vi "Attocube Main.vi"() -> ()   [LabVIEW 2013]
panel:
  out "last move time":timestamp
  out "axis 1:\nCurrent position [µm/°/m°] 2":dbl(knob) scale=65.0..270.0 scale format="%#_3p"
  out "axis 1:\nCurrent position (°)":dbl format="%.4f"
  in  "set static amplitude\nwhen moving":bool
  in  "static amplitude (mV)":dbl=2.0 min=0.001 max=2.0 format="%#_13g"
  in  "both axes: Output":bool caption="both axes:\nOutput"
  in  "axis 2:\nStop moving":bool
  in  "axis 1:\nStop moving":bool
  in  "Remote mode":bool
  in  "axis 2:\nstop detection":bool
  in  "axis 1:\nstop detection":bool
  in  "axis 2:\nOutput":bool
  in  "axis 1:\ncontrol mode":enum16{"speed", "amplitude", "step size"}(ring)=enum."amplitude"
  in  "axis 2:\ncontrol mode":enum16{"speed", "amplitude", "step size"}(ring)=enum."amplitude"
  in  "axis 1:\nOutput":bool
  out "axis 2:\nStepWidth":i32=38 format="%.0fnm"
  out "axis 1:\nStepWidth":i32 format="%.0fnm"
  out "axis 2:\nspeed (°/s)":i32=31
  out "axis 1:\nspeed (°/s)":i32
  out "axis 2:\nCapacitance":i32=2486 format="%.0fnF"
  out "axis 1:\nCapacitance":i32=2534 format="%.0fnF"
  in  "axis 2:\ncap. measure":bool
  in  "axis 1:\ncap. measure":bool
  out "axis 2:\nCurrent position [µm/°/m°] 2":dbl(knob) scale=5.0..320.0
  in  "axis 2:\nFrequency [Hz]":i32=800 min=0 max=20000 format="%.0fHz"
  in  "axis 1:\nFrequency [Hz]":i32=800 min=0 max=20000 format="%.0fHz"
  in  "axis 2:\nDCLevel [V]":dbl min=0.0 max=140.0 step=0.001 format="%.3f"
  in  "axis 1:\nDCLevel [V]":dbl min=0.0 max=140.0 step=0.001 format="%.3f"
  in  "axis 2:\nAmplitude [V]":dbl=35.0 min=0.0 max=150.0 format="%.3gV"
  in  "axis 1:\nAmplitude [V]":dbl=40.0 min=0.0 max=150.0 format="%.3gV"
  in  "axis 2:\ncontinuous back":bool
  in  "axis 2:\ncontinuous fwd":bool
  in  "axis 1:\ncontinuous back":bool
  in  "axis 1:\ncontinuous fwd":bool
  in  "axis 2:\nsingle step fwd":bool
  in  "axis 2:\nsingle step back":bool
  in  "axis 1:\nsingle step back":bool
  in  "axis 1:\nsingle step fwd":bool
  in  "axis 2:\nsp position °":dbl=78.5 min=5.0 max=320.0 format="%.4g"
  in  "axis 2:\nsp rot count":i32
  in  "axis 1:\nsp rot count":i32
  in  "axis 1:\nsp position °":dbl=167.0 min=65.0 max=270.0 format="%.4g"
  in  "axis 2:\nAbsolute":bool
  in  "axis 2:\nRelative":bool
  in  "axis 1:\nRelative":bool
  in  "axis 1:\nAbsolute":bool
  in  "axis 1: \nTarget GND":bool
  in  "axis 1:\nSingle Circle Mode":bool
  in  "axis 2:\nSingle Circle Mode":bool
  in  "axis 2: \nTarget GND":bool
  out "axis 2:\npositioner status":T1
  out "axis 2:\nCurrent position (°)":dbl format="%.4f"
  out "axis 2:\nrot. count":i32
  out "axis 1:\npositioner status":T1
  out "axis 1:\nrot. count":i32
  out "handle":i32=5
  in  "OK":bool
  # "Axis 1: large axis"
  # "Axis 2: small axis"
  # "Notes: \n\n***Switch controller to ground (output=false) before connecting the rotator and while cooling down/warming up***\n\nAxis 1 (large axis): Position is limited by physical stops to angles from 65° to 270°\n\nAxis 2 (small axis): Encoded positions are limited to angles from 5° to 320°, not physically limited to one rotation.  Keep single circle mode OFF to limit the rotation count to zero and protect the wiring from over-rotating.\n\nStatic Amplitude: Sets the voltage applied to the resitive readout system.  Range: 0.001 V to 2V.  Higher voltages enhace the sensitivity but lower voltages minimize heat dissipation for low temperature applications.\n\nAbsolute: positioner travels from its current position to      the target position.\n\nTarget Ground: positioner will be grounded when the target position is reached.\n\nSingle circle mode: If OFF absolute and relative positioning are only allowed up to a full circle, keeps rot count at zero.\n\nOutput: When checked, the repective axis output is enabled.  Deactivating sets the axis to GND\n\nControl mode: \n     amplitude: individual steps of the piezo are definied by        the amplitude.  Driven in open-loop mode, travel speed and step width may vary\n     speed: feedback enables a constant travel speed by closed-loop control of the amplitude and frequency.  Speed is set by adjusting the amplitude and/or frequency values.\n     step width: Step size in controlled to a constant value.  Amplitude is closed-loop controlled.  Step width is set by adjusting the amplitude"
  # "Automatic Positioning"
  # "Automatic Positioning"
  # "Manual Positioning"
  # "Manual Positioning"
  # "Move Single Step"
  # "Move Single Step"
  # "Move Continuous"
  # "Move Continuous"
  # "Capacitance Measurement"
  # "Capacitance Measurement"
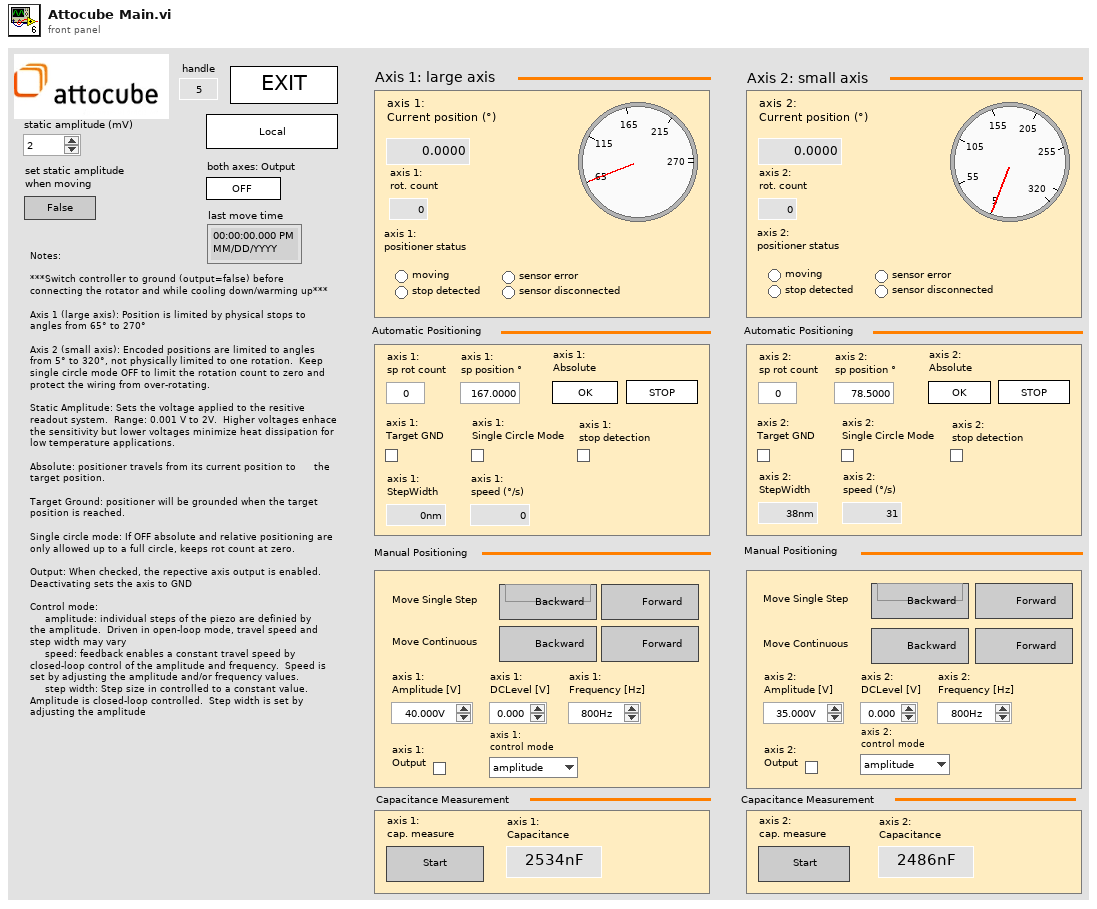
[diagram p1: front panel]
types:
  T1 = cluster{"moving":bool, "stop detected":bool, "sensor error":bool, "sensor disconnected":bool}
  T2 = enum32{"invalid app kind", "Development System", "Run Time System", "Student Edition", "Embedded LabVIEW", "Evaluation", "Custom"}
  T3 = enum32{"Invalid", "Standard", "Closed", "Hidden", "Minimized", "Maximized"}
  T4 = cluster{"axis 1: Absolute":bool, "axis 2: Absolute":bool, "axis 1: Stop moving":bool, "axis 2: Stop moving":bool, "axis 1: Output":bool, "axis 2: Output":bool, "set static amplitude\nwhen moving":bool}
  T5 = cluster{"axis 1: Amplitude [V]":dbl, "axis 2: Amplitude [V]":dbl, "axis 1: DCLevel [V]":dbl, "axis 2: DCLevel [V]":dbl, "axis 1: Frequency [Hz]":dbl, "axis 2: Frequency [Hz]":dbl, "axis 1: sp position °":dbl, "axis 2: sp position °":dbl, "axis 1: sp rot count":dbl, "axis 2: sp rot count":dbl}
  T6 = cluster{"error ":bool, "error number":i32, "error code":string}
  T7 = cluster{"Core":cluster{"Current VI Reference":refnum<vi>, "Close Panel on Exit?":bool}, "handle":i32}
  T8 = cluster{"Current VI Reference":refnum<vi>, "Close Panel on Exit?":bool}
  T9 = cluster{"axis 1: Current position (°)":dbl, "axis 2: Current position (°)":dbl, "axis 1: rot. count":dbl, "axis 2: rot. count":dbl, "axis 1: StepWidth":dbl, "axis 2: StepWidth":dbl, "axis 1: speed (°/s)":dbl, "axis 2: speed (°/s)":dbl, "axis 1: positioner status":cluster{"moving":bool, "stop detected":bool, "sensor error":bool, "sensor disconnected":bool}, "axis 2: positioner status":cluster{"moving":bool, "stop detected":bool, "sensor error":bool, "sensor disconnected":bool}}
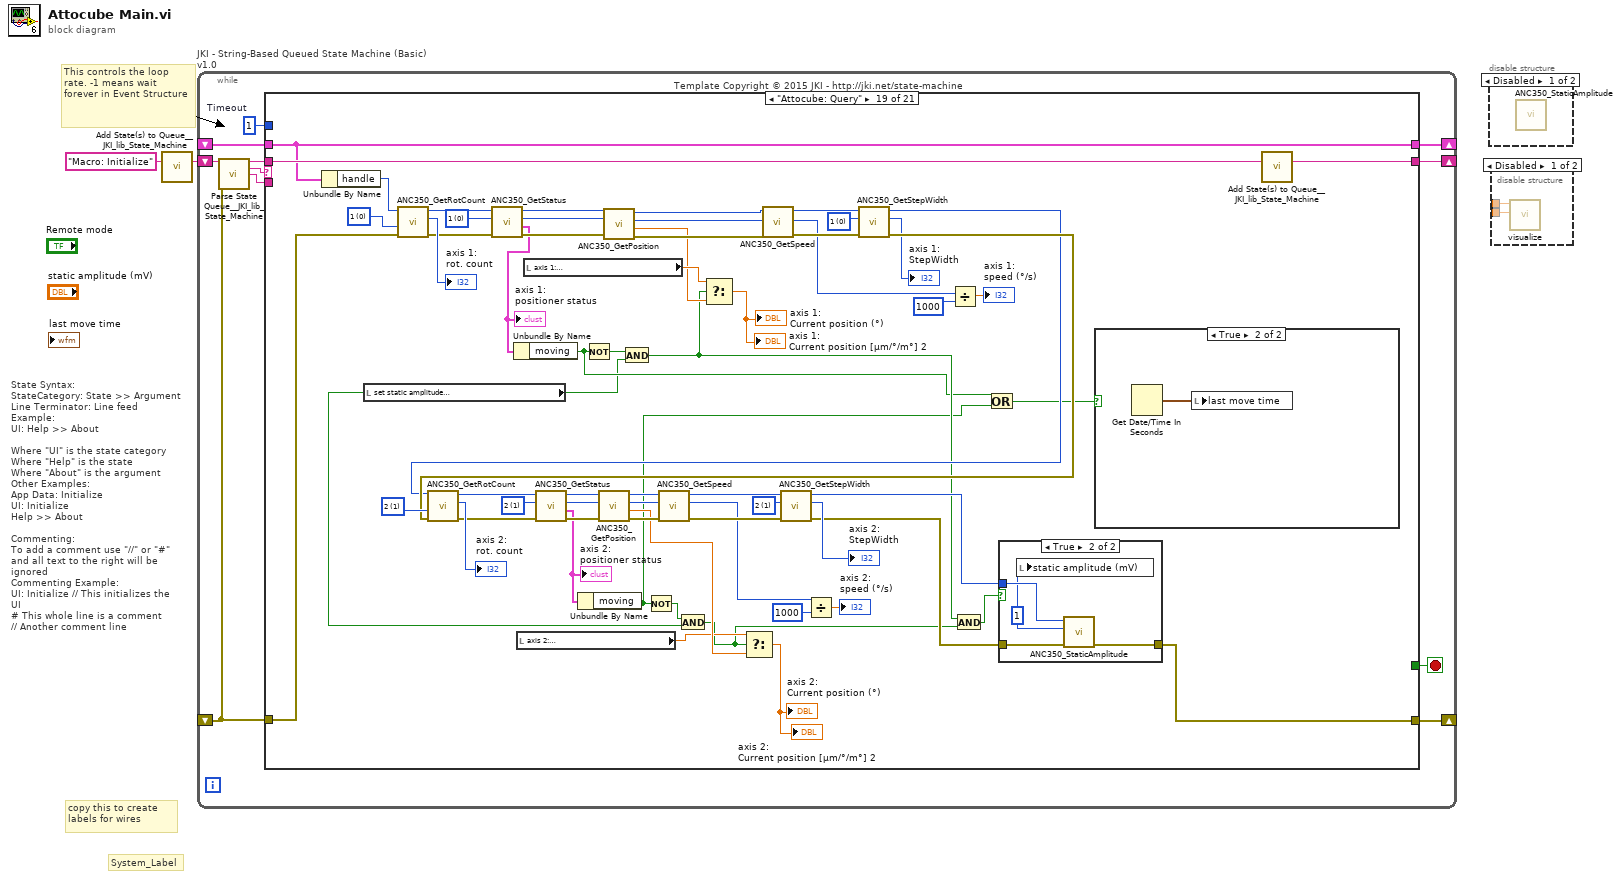
[diagram p0: block diagram]
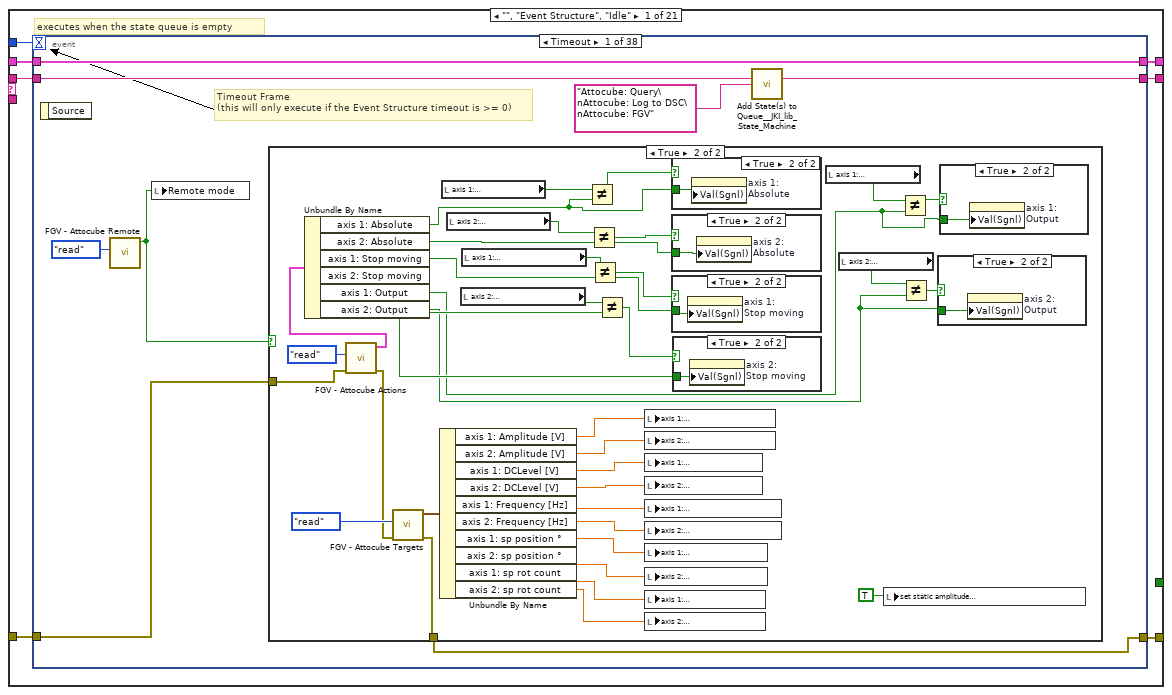
[diagram p4: hidden frame]
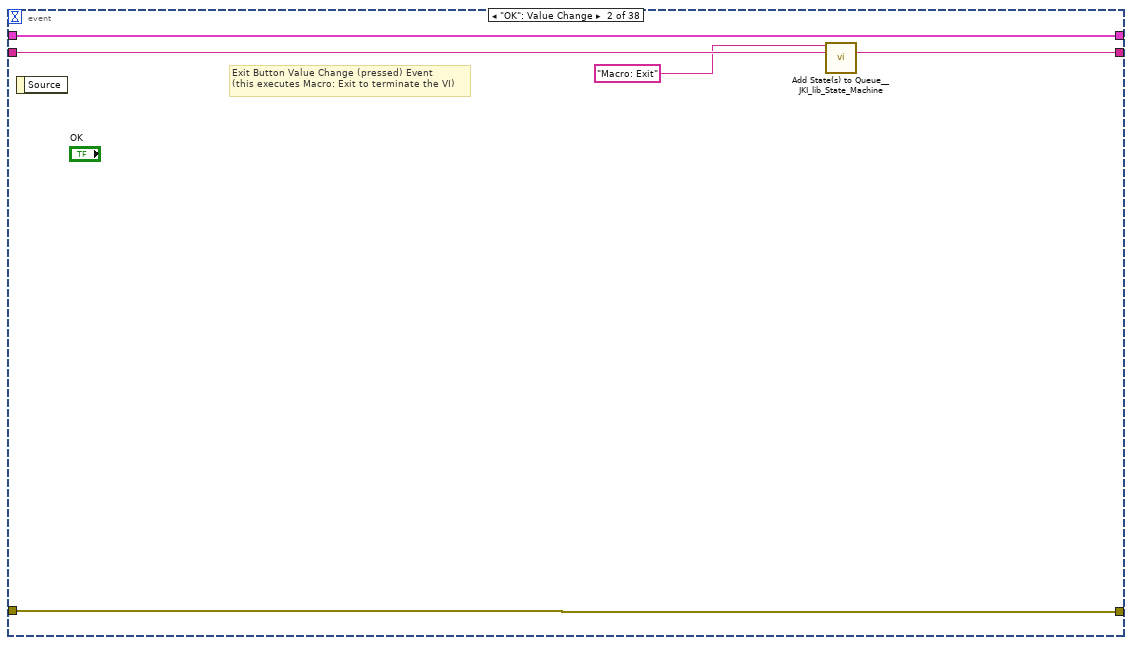
[diagram p12: hidden frame]
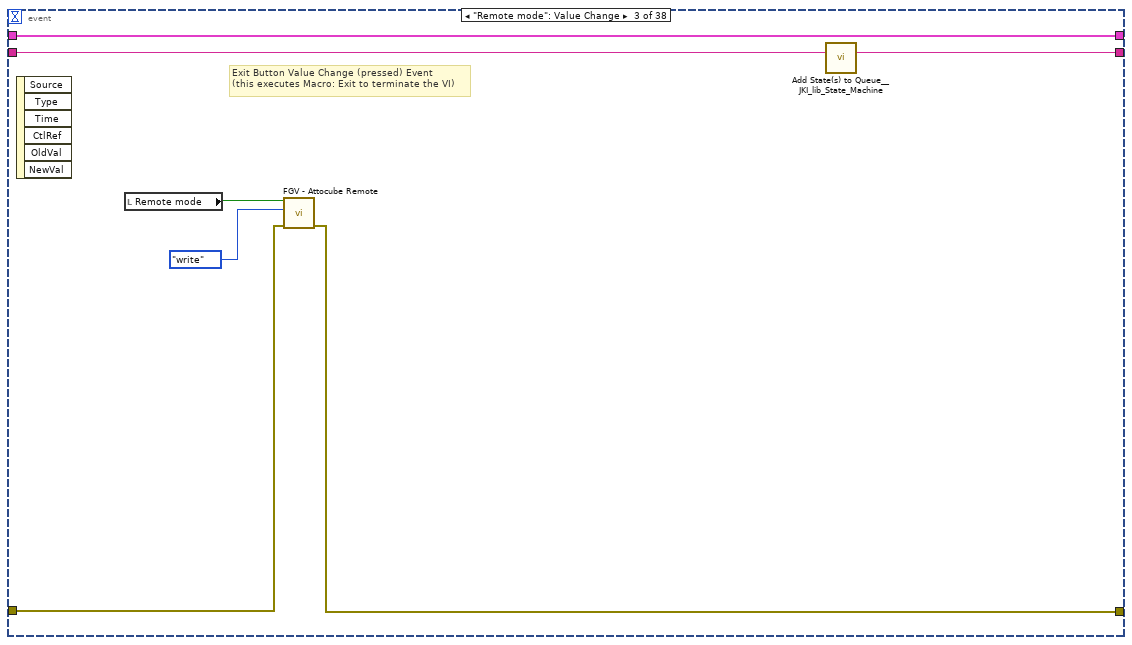
[diagram p13: hidden frame]
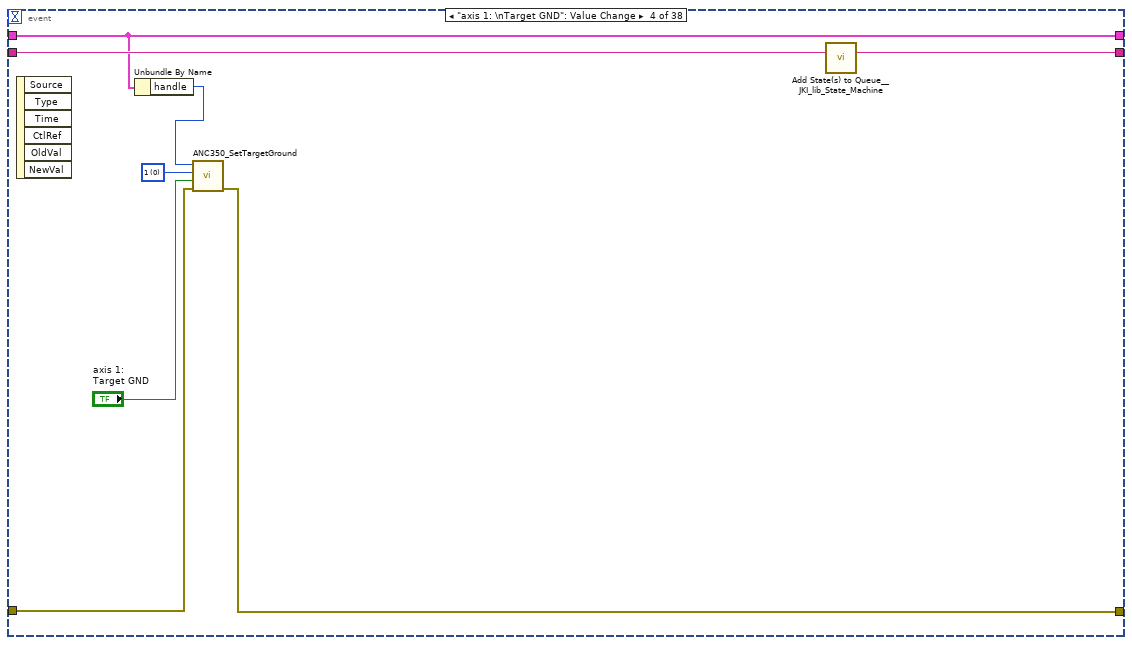
[diagram p14: hidden frame]
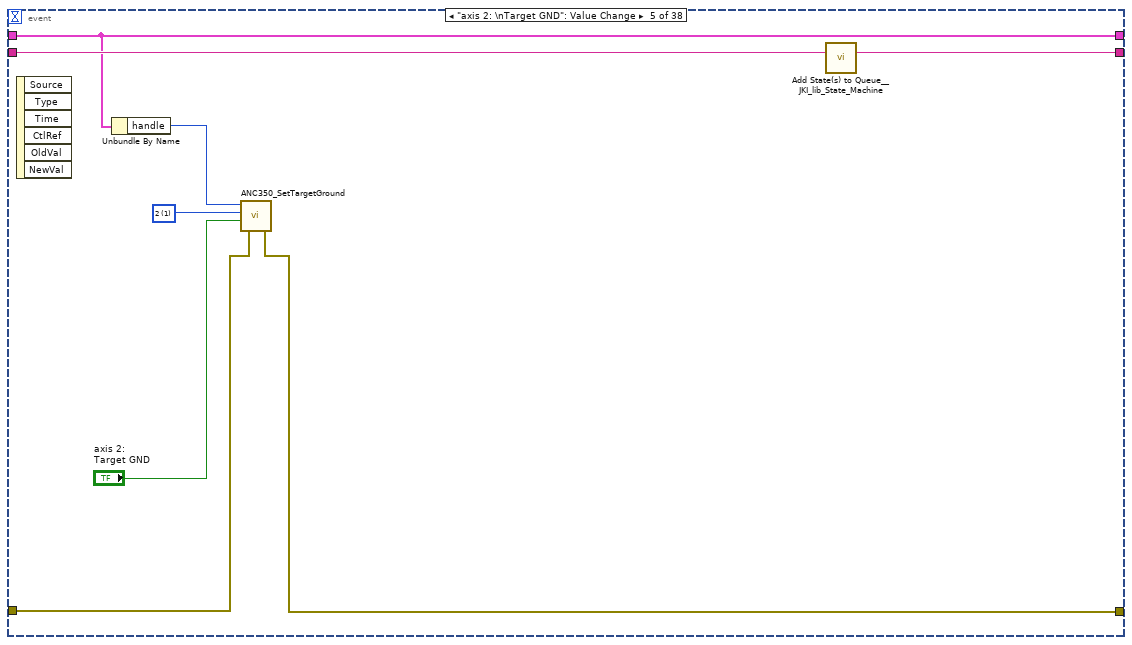
[diagram p15: hidden frame]
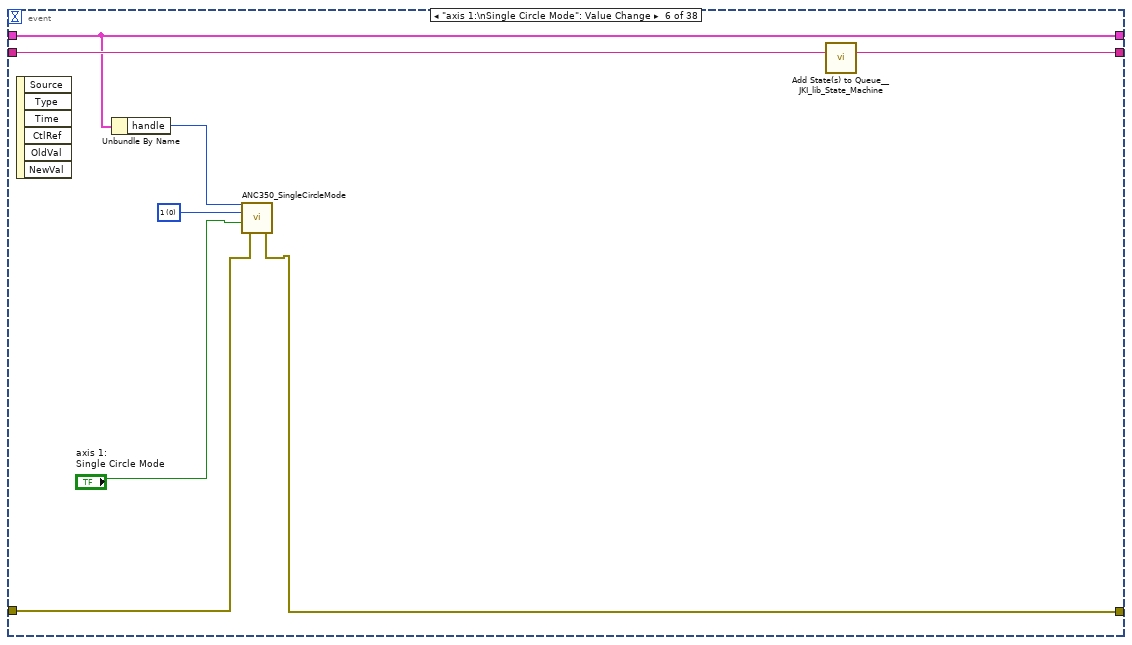
[diagram p16: hidden frame]
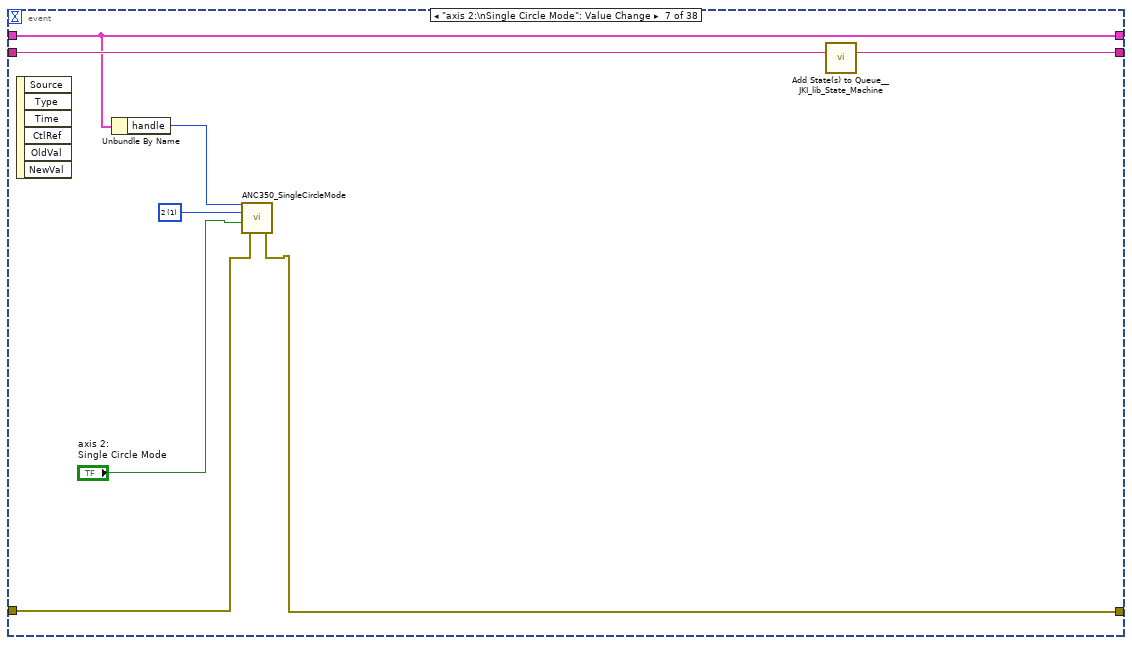
[diagram p17: hidden frame]
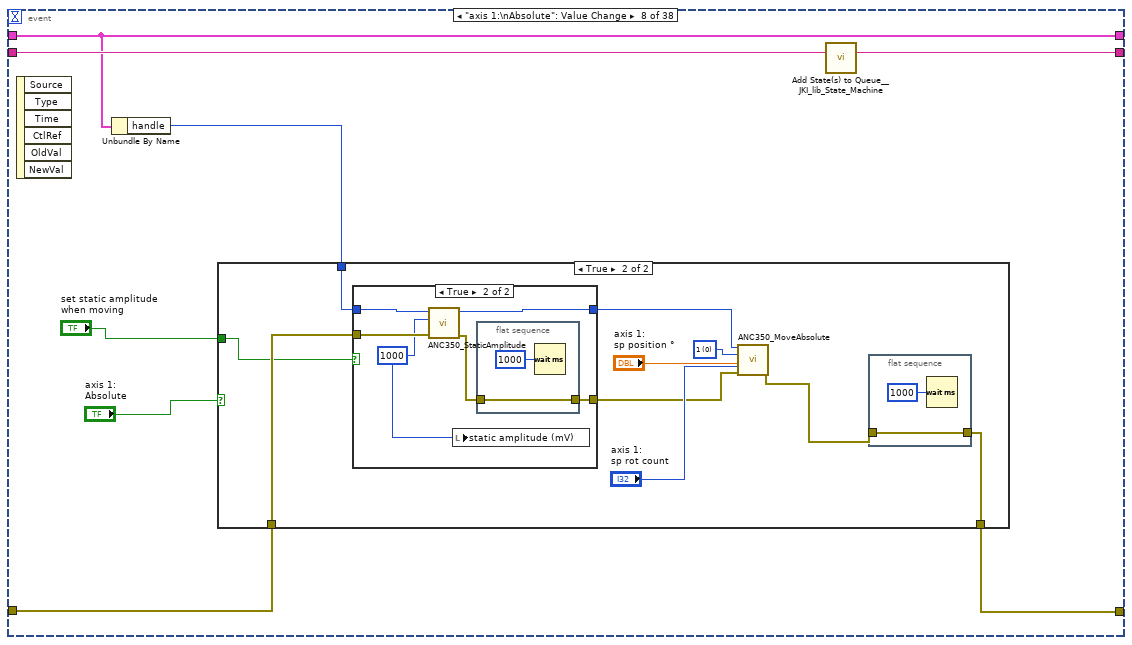
[diagram p18: hidden frame]
diagram:
  # "State Syntax:\nStateCategory: State >> Argument\nLine Terminator: Line feed\nExample:\nUI: Help >> About\n\nWhere \"UI\" is the state category\nWhere \"Help\" is the state\nWhere \"About\" is the argument\nOther Examples:\nApp Data: Initialize\nUI: Initialize\nHelp >> About\n\nCommenting:\nTo add a comment use \"//\" or \"#\" and all text to the right will be ignored\nCommenting Example:\nUI: Initialize // This initializes the UI\n# This whole line is a comment\n// Another comment line"
  # "copy this to create labels for wires"
  # "This controls the loop rate. -1 means wait forever in Event Structure"
  # "System_Label"
  n1 = call <vilib>:"Add State(s) to Queue__JKI_lib_State_Machine.vi"("State(s) in (\"\")"="Macro: Initialize") -> ("States Out"=w2:string)  [unwired: 14 in]
  n2 = while "JKI - String-Based Queued State Machine (Basic) v1.0" {
    shift-right: [w7] -> _
    shift-left: _ -> [w6]
    shift-right: [w3] -> _
    shift-left: _ -> [w4]
    shift-right: [w9] -> _
    shift-left: w2 -> [w10]
    stop <- w8 stop-if-true
    w5 = 1  # Timeout
    # "Template Copyright © 2015 JKI - http://jki.net/state-machine"
    n3 = call <vilib>:"Parse State Queue__JKI_lib_State_Machine.vi"("State Queue"=w10, "Error In (no error)"=w4) -> ("Remaining States"=w12:string, "Current State"=w13:string, "Arguments"=w11:string)  [unwired: 11 in]
    n4 = case shown="\"Attocube: Query\"" w13 {
      selector: w13 -> [_ _ w500 _ _ _ _ _ _ _ _ _ _ _ _ _ _ _ _ _ _]
      tunnel: w12 -> [w20 w499 w504 w522 w528 w533 w537 w543 w549 w553 w564 w575 w586 w612 w617 w643 w647 w655 w721 w782 w831]
      tunnel: w11 -> [_ _ _ _ _ _ _ _ _ _ _ w570 w580 _ _ _ _ _ _ _ _]
      tunnel: w6 -> [w18 w496 w502 w513 w525 w531 w534 _ w544 w550 w562 w573 w582 w609 w614 w641 w644 w653 w719 w780 w829]
      tunnel: w4 -> [w16 w497 w505 w519 w524 w530 w535 w540 w546 w551 w561 w572 w584 w610 w615 w631 w645 _ w718 w735 w824]
      tunnel: [w19 w498 w503 w521 w527 w532 w536 w542 w548 w552 w563 w574 w585 w611 w616 w642 w646 w654 w720 w781 w830] -> w9
      tunnel: [_ _ _ _ _ TRUE _ _ _ _ _ _ _ _ _ _ _ _ _ _ _] -> w8
      tunnel: [w15 w496 w502 w520 w525 w531 w534 w541 w544 w550 w562 w573 w582 w609 w614 w641 w644 w652 w719 w780 w829] -> w7
      tunnel: w5 -> [w14 _ _ _ _ _ _ _ _ _ _ _ _ _ _ _ _ _ _ _ _]
      tunnel: [w17 w497 w506 w519 errorcluster {"status"=FALSE, "code"=0, "source"=""} ("error out") w530 w535 w540 w545 w551 w561 w571 w583 w610 w615 w634 w645 w649 w668 w735 w787] -> w3
      frame "", "Event Structure", "Idle" {
        # "executes when the state queue is empty"
        n5 = event shown="[0] Timeout" {
          selector: _ -> [_ _ _ _ _ _ _ _ _ _ _ _ _ _ _ _ _ _ _ _ _ _ _ _ _ _ _ _ _ _ _ _ _ _ _ _ _ _]
          dyn-events: _ -> [_ _ _ _ _ _ _ _ _ _ _ _ _ _ _ _ _ _ _ _ _ _ _ _ _ _ _ _ _ _ _ _ _ _ _ _ _ _]
          timeout: w14 -> [_ _ _ _ _ _ _ _ _ _ _ _ _ _ _ _ _ _ _ _ _ _ _ _ _ _ _ _ _ _ _ _ _ _ _ _ _ _]
          tunnel: w20 -> [w28 w76 w83 w91 w99 w107 w115 w123 w154 w184 w198 w212 w225 w238 w251 w264 w280 w296 w312 w329 w337 w345 w353 w361 w369 w377 w391 w405 w413 w421 w429 w437 w445 w453 w466 w476 w484 w495]
          tunnel: [w27 w75 w82 w90 w98 w106 w114 w122 w153 w183 w197 w211 w224 w237 w250 w263 w279 w295 w311 w328 w336 w344 w352 w360 w368 w376 w390 w404 w412 w420 w428 w436 w444 w452 w465 w475 w483 w494] -> w19
          tunnel: w18 -> [w26 w73 w81 w89 w97 w105 w113 w121 w152 w182 w196 w210 w223 w236 w249 w262 w278 w294 w310 w327 w335 w343 w351 w359 w367 w375 w389 w403 w411 w419 w427 w435 w443 w451 w464 w474 w482 w492]
          tunnel: [w21 w74 w77 w84 w94 w100 w110 w116 w149 w179 w193 w207 w220 w233 w246 w259 w275 w291 w307 w322 w331 w338 w347 w354 w363 w371 w385 w399 w407 w416 w424 w431 w439 w447 w460 w473 w479 w493] -> w17
          tunnel: w16 -> [w22 w74 w78 w85 w95 w101 w111 w119 w150 w180 w194 w208 w221 w234 w247 w260 w276 w292 w308 w323 w332 w339 w348 w355 w364 w372 w386 w400 w408 w417 w425 w432 w440 w448 w461 w473 w480 w493]
          tunnel: [w26 w73 w81 w89 w97 w105 w113 w121 w152 w182 w196 w210 w223 w236 w249 w262 w278 w294 w310 w327 w335 w343 w351 w359 w367 w375 w389 w403 w411 w419 w427 w435 w443 w451 w464 w474 w482 w492] -> w15
          event Timeout {
            # "Timeout Frame\n(this will only execute if the Event Structure timeout is >= 0)"
            n6 = event-data() -> ()  [unwired: 1 in, 1 out]
            n7 = call "FGV - Attocube Remote.vi"("Function"=enum16{"write", "read"}."read") -> ("Attocube Remote"=w23:bool)  [unwired: 5 in, 1 out]
            n8 = local write "Remote mode"(w23) -> ()
            n9 = case shown="True" w23 {
              tunnel: w22 -> [w29 w39]
              tunnel: [w29 w37] -> w21
              frame False {
              }
              frame True {
                n10 = call "FGV - Attocube Actions.vi"("error in"=w39, "Function"=enum16{"write", "read"}."read") -> ("error out"=w38:errorcluster, "Actions OUT"=w64:T4)  [unwired: 4 in]
                n11 = Unbundle By Name(w64) -> ("axis 1: Absolute"=w58:bool, "axis 2: Absolute"=w57:bool, "axis 1: Stop moving"=w53:bool, "axis 2: Stop moving"=w52:bool, "axis 1: Output"=w33:bool, "axis 2: Output"=w30:bool)
                n12 = call "FGV - Attocube Targets.vi"("error in"=w38, "Function"=enum16{"write", "read"}."read") -> ("error out"=w37:errorcluster, "Targets Out"=w50:T5)  [unwired: 4 in]
                n13 = Unbundle By Name(w50) -> ("axis 1: Amplitude [V]"=w49:dbl, "axis 2: Amplitude [V]"=w48:dbl, "axis 1: DCLevel [V]"=w47:dbl, "axis 2: DCLevel [V]"=w46:dbl, "axis 1: Frequency [Hz]"=w45:dbl, "axis 2: Frequency [Hz]"=w44:dbl, "axis 1: sp position °"=w43:dbl, "axis 2: sp position °"=w42:dbl, "axis 1: sp rot count"=w41:dbl, "axis 2: sp rot count"=w40:dbl)
                n14 = local read "axis 1:\nAbsolute"() -> (w63:bool)
                n15 = local read "axis 2:\nAbsolute"() -> (w62:bool)
                n16 = local read "axis 2:\nStop moving"() -> (w60:bool)
                n17 = local read "axis 1:\nStop moving"() -> (w61:bool)
                n18 = Not Equal?(x=w63, y=w58) -> (x != y?=w59:bool)
                n19 = Not Equal?(x=w62, y=w57) -> (x != y?=w56:bool)
                n20 = Not Equal?(x=w61, y=w53) -> (x != y?=w55:bool)
                n21 = Not Equal?(x=w60, y=w52) -> (x != y?=w54:bool)
                n22 = local write "axis 1:\nAmplitude [V]"(w49) -> ()
                n23 = local write "axis 2:\nAmplitude [V]"(w48) -> ()
                n24 = local write "axis 1:\nDCLevel [V]"(w47) -> ()
                n25 = local write "axis 2:\nDCLevel [V]"(w46) -> ()
                n26 = local write "axis 1:\nFrequency [Hz]"(w45) -> ()
                n27 = local write "axis 2:\nFrequency [Hz]"(w44) -> ()
                n28 = local write "axis 1:\nsp position °"(w43) -> ()
                n29 = local write "axis 2:\nsp position °"(w42) -> ()
                n30 = local write "axis 1:\nsp rot count"(w41) -> ()
                n31 = local write "axis 2:\nsp rot count"(w40) -> ()
                n32 = case shown="True" w59 {
                  tunnel: w58 -> [_ w71]
                  frame False {
                  }
                  frame True {
                    n33 = property on="axis 1:\nAbsolute" class="Bool (strict)"("Val(Sgnl)"=w71) -> ()  [unwired: 2 in, 2 out]
                  }
                }
                n34 = case shown="True" w56 {
                  tunnel: w57 -> [_ w70]
                  frame False {
                  }
                  frame True {
                    n35 = property on="axis 2:\nAbsolute" class="Bool (strict)"("Val(Sgnl)"=w70) -> ()  [unwired: 2 in, 2 out]
                  }
                }
                n36 = case shown="True" w55 {
                  tunnel: w53 -> [_ w69]
                  frame False {
                  }
                  frame True {
                    n37 = property on="axis 1:\nStop moving" class="Bool (strict)"("Val(Sgnl)"=w69) -> ()  [unwired: 2 in, 2 out]
                  }
                }
                n38 = case shown="True" w54 {
                  tunnel: w52 -> [_ w68]
                  frame False {
                  }
                  frame True {
                    n39 = property on="axis 2:\nStop moving" class="Bool (strict)"("Val(Sgnl)"=w68) -> ()  [unwired: 2 in, 2 out]
                  }
                }
                n40 = local read "axis 1:\nOutput"() -> (w34:bool)
                n41 = local read "axis 2:\nOutput"() -> (w31:bool)
                n42 = local write "set static amplitude\nwhen moving"(TRUE) -> ()
                n43 = Not Equal?(x=w34, y=w33) -> (x != y?=w35:bool)
                n44 = Not Equal?(x=w31, y=w30) -> (x != y?=w32:bool)
                n45 = case shown="True" w32 {
                  tunnel: w30 -> [_ w66]
                  frame False {
                  }
                  frame True {
                    n46 = property on="axis 2:\nOutput" class="Bool (strict)"("Val(Sgnl)"=w66) -> ()  [unwired: 2 in, 2 out]
                  }
                }
                n47 = case shown="True" w35 {
                  tunnel: w33 -> [_ w67]
                  frame False {
                  }
                  frame True {
                    n48 = property on="axis 1:\nOutput" class="Bool (strict)"("Val(Sgnl)"=w67) -> ()  [unwired: 2 in, 2 out]
                  }
                }
              }
            }
            n49 = call <vilib>:"Add State(s) to Queue__JKI_lib_State_Machine.vi"("State(s) in (\"\")"=w28, "State(s) at Back (\"\")"="Attocube: Query\nAttocube: Log to DSC\nAttocube: FGV" ("State(s) at Back (\"\")")) -> ("States Out"=w27:string)  [unwired: 13 in]
          }
          event "OK": Value Change {
            # "Exit Button Value Change (pressed) Event\n(this executes Macro: Exit to terminate the VI)"
            n50 = event-data() -> ()  [unwired: 1 in, 1 out]
            n51 = call <vilib>:"Add State(s) to Queue__JKI_lib_State_Machine.vi"("State(s) in Front (\"\")"="Macro: Exit", "State(s) in (\"\")"=w76) -> ("States Out"=w75:string)  [unwired: 13 in]
          }
          event "Remote mode": Value Change {
            # "Exit Button Value Change (pressed) Event\n(this executes Macro: Exit to terminate the VI)"
            n52 = event-data() -> ()  [unwired: 1 in, 6 out]
            n53 = local read "Remote mode"() -> (w80:bool)
            n54 = call "FGV - Attocube Remote.vi"("error in"=w78, "Function"=enum16{"write", "read"}."write", "Attocube Remote"=w80) -> ("error out"=w77:errorcluster)  [unwired: 3 in, 1 out]
            n55 = call <vilib>:"Add State(s) to Queue__JKI_lib_State_Machine.vi"("State(s) in (\"\")"=w83) -> ("States Out"=w82:string)  [unwired: 14 in]
          }
          event "axis 1: \nTarget GND": Value Change {
            w87 = u8 0 items=["1", "2", "3", "4", "5", "6", "7", "8", "9"] ("axis no")
            n56 = event-data() -> ()  [unwired: 1 in, 6 out]
            n57 = Unbundle By Name(w89) -> ("handle"=w88:i32)
            n58 = call "ANC350_SetTargetGround.vi"("error in"=w85, "PositionerAcIn"="axis 1: \nTarget GND", "axis no"=w87, "device handle"=w88) -> ("error out"=w84:T6)  [unwired: 2 in, 1 out]
            n59 = call <vilib>:"Add State(s) to Queue__JKI_lib_State_Machine.vi"("State(s) in (\"\")"=w91) -> ("States Out"=w90:string)  [unwired: 14 in]
          }
          event "axis 2: \nTarget GND": Value Change {
            w93 = u8 1 items=["1", "2", "3", "4", "5", "6", "7", "8", "9"] ("axis no")
            n60 = event-data() -> ()  [unwired: 1 in, 6 out]
            n61 = Unbundle By Name(w97) -> ("handle"=w96:i32)
            n62 = call "ANC350_SetTargetGround.vi"("error in"=w95, "PositionerAcIn"="axis 2: \nTarget GND", "axis no"=w93, "device handle"=w96) -> ("error out"=w94:T6)  [unwired: 2 in, 1 out]
            n63 = call <vilib>:"Add State(s) to Queue__JKI_lib_State_Machine.vi"("State(s) in (\"\")"=w99) -> ("States Out"=w98:string)  [unwired: 14 in]
          }
          event "axis 1:\nSingle Circle Mode": Value Change {
            w103 = u8 0 items=["1", "2", "3", "4", "5", "6", "7", "8", "9"] ("axis no")
            n64 = event-data() -> ()  [unwired: 1 in, 6 out]
            n65 = Unbundle By Name(w105) -> ("handle"=w104:i32)
            n66 = call "ANC350_SingleCircleMode.vi"("error in"=w101, "enable"="axis 1:\nSingle Circle Mode", "axis no"=w103, "device handle"=w104) -> ("error out"=w100:T6)  [unwired: 2 in, 1 out]
            n67 = call <vilib>:"Add State(s) to Queue__JKI_lib_State_Machine.vi"("State(s) in (\"\")"=w107) -> ("States Out"=w106:string)  [unwired: 14 in]
          }
          event "axis 2:\nSingle Circle Mode": Value Change {
            w108 = u8 1 items=["1", "2", "3", "4", "5", "6", "7", "8", "9"] ("axis no")
            n68 = event-data() -> ()  [unwired: 1 in, 6 out]
            n69 = Unbundle By Name(w113) -> ("handle"=w112:i32)
            n70 = call "ANC350_SingleCircleMode.vi"("error in"=w111, "enable"="axis 2:\nSingle Circle Mode", "axis no"=w108, "device handle"=w112) -> ("error out"=w110:T6)  [unwired: 2 in, 1 out]
            n71 = call <vilib>:"Add State(s) to Queue__JKI_lib_State_Machine.vi"("State(s) in (\"\")"=w115) -> ("States Out"=w114:string)  [unwired: 14 in]
          }
          event "axis 1:\nAbsolute": Value Change {
            n72 = event-data() -> ()  [unwired: 1 in, 6 out]
            n73 = Unbundle By Name(w121) -> ("handle"=w120:i32)
            n74 = case shown="True" "axis 1:\nAbsolute" {
              tunnel: w120 -> [_ w131]
              tunnel: w119 -> [w124 w129]
              tunnel: "set static amplitude\nwhen moving" -> [_ w127]
              tunnel: [w124 w125] -> w116
              frame False {
              }
              frame True {
                w134 = u8 0 items=["1", "2", "3", "4", "5", "6", "7", "8", "9"] ("axis no")
                n75 = case shown="True" w127 {
                  tunnel: w131 -> [w138 w144]
                  tunnel: [w138 w143] -> w130
                  tunnel: w129 -> [w137 w142]
                  tunnel: [w137 w140] -> w128
                  frame False {
                  }
                  frame True {
                    w139 = 1000 ("static amplitude")
                    n76 = call "ANC350_StaticAmplitude.vi"("error in"=w142, "static amplitude"=w139, "device handle"=w144) -> ("error out"=w141:T6, "device handle Out"=w143:i32)  [unwired: 3 in]
                    n77 = local write "static amplitude (mV)"(w139) -> ()
                    n78 = flat-sequence {
                      tunnel: [w146] -> w140
                      tunnel: w141 -> [w146]
                      frame #0 {
                        n79 = Wait (ms)(milliseconds to wait=u32 1000) -> ()  [unwired: 1 out]
                      }
                    }
                  }
                }
                n80 = call "ANC350_MoveAbsolute.vi"("device handle"=w130, "axis no"=w134, "absoluteposition [µm/°/m°]"="axis 1:\nsp position °", "rot count"="axis 1:\nsp rot count", "error in"=w128) -> ("error out"=w126:T6)  [unwired: 9 in, 1 out]
                n81 = flat-sequence {
                  tunnel: [w136] -> w125
                  tunnel: w126 -> [w136]
                  frame #0 {
                    n82 = Wait (ms)(milliseconds to wait=u32 1000) -> ()  [unwired: 1 out]
                  }
                }
              }
            }
            n83 = call <vilib>:"Add State(s) to Queue__JKI_lib_State_Machine.vi"("State(s) in (\"\")"=w123) -> ("States Out"=w122:string)  [unwired: 14 in]
          }
          event "axis 2:\nAbsolute": Value Change {
            n84 = event-data() -> ()  [unwired: 1 in, 6 out]
            n85 = local read "set static amplitude\nwhen moving"() -> (w147:bool)
            n86 = Unbundle By Name(w152) -> ("handle"=w151:i32)
            n87 = case shown="True" "axis 2:\nAbsolute" {
              tunnel: w151 -> [_ w162]
              tunnel: w150 -> [w155 w160]
              tunnel: [w155 w156] -> w149
              tunnel: w147 -> [_ w158]
              frame False {
              }
              frame True {
                w165 = u8 1 items=["1", "2", "3", "4", "5", "6", "7", "8", "9"] ("axis no")
                n88 = case shown="True" w158 {
                  tunnel: w162 -> [w169 w175]
                  tunnel: [w169 w174] -> w161
                  tunnel: w160 -> [w168 w173]
                  tunnel: [w168 w171] -> w159
                  frame False {
                  }
                  frame True {
                    w170 = 1000 ("static amplitude")
                    n89 = local write "static amplitude (mV)"(w170) -> ()
                    n90 = call "ANC350_StaticAmplitude.vi"("error in"=w173, "static amplitude"=w170, "device handle"=w175) -> ("error out"=w172:T6, "device handle Out"=w174:i32)  [unwired: 3 in]
                    n91 = flat-sequence {
                      tunnel: [w177] -> w171
                      tunnel: w172 -> [w177]
                      frame #0 {
                        n92 = Wait (ms)(milliseconds to wait=u32 1000) -> ()  [unwired: 1 out]
                      }
                    }
                  }
                }
                n93 = call "ANC350_MoveAbsolute.vi"("device handle"=w161, "axis no"=w165, "absoluteposition [µm/°/m°]"="axis 2:\nsp position °", "rot count"="axis 2:\nsp rot count", "error in"=w159) -> ("error out"=w157:T6)  [unwired: 9 in, 1 out]
                n94 = flat-sequence {
                  tunnel: [w167] -> w156
                  tunnel: w157 -> [w167]
                  frame #0 {
                    n95 = Wait (ms)(milliseconds to wait=u32 1000) -> ()  [unwired: 1 out]
                  }
                }
              }
            }
            n96 = call <vilib>:"Add State(s) to Queue__JKI_lib_State_Machine.vi"("State(s) in (\"\")"=w154) -> ("States Out"=w153:string)  [unwired: 14 in]
          }
          event "axis 1:\nRelative": Value Change {
            n97 = event-data() -> ()  [unwired: 1 in, 6 out]
            n98 = disable-structure shown="Disabled" {
              frame Disabled {
              }
              frame Enabled {
              }
            }
            n99 = Unbundle By Name(w182) -> ("handle"=w181:i32)
            n100 = case shown="True" FALSE {
              tunnel: w181 -> [_ w191]
              tunnel: w180 -> [w185 w189]
              tunnel: [w185 w186] -> w179
              frame False {
              }
              frame True {
                w190 = u8 0 items=["1", "2", "3", "4", "5", "6", "7", "8", "9"] ("axis no")
                n101 = local read "axis 1:\nsp position °"() -> (w188:dbl)
                n102 = local read "axis 1:\nsp rot count"() -> (w187:i32)
                n103 = call "ANC350_MoveRelative.vi"("device handle"=w191, "axis no"=w190, "distance [µm/°/m°]"=w188, "rot count"=w187, "error in"=w189) -> ("error out"=w186:T6)  [unwired: 9 in, 1 out]
              }
            }
            n104 = call <vilib>:"Add State(s) to Queue__JKI_lib_State_Machine.vi"("State(s) in (\"\")"=w184) -> ("States Out"=w183:string)  [unwired: 14 in]
          }
          event "axis 2:\nRelative": Value Change {
            n105 = event-data() -> ()  [unwired: 1 in, 6 out]
            n106 = disable-structure shown="Disabled" {
              frame Disabled {
              }
              frame Enabled {
              }
            }
            n107 = Unbundle By Name(w196) -> ("handle"=w195:i32)
            n108 = case shown="True" FALSE {
              tunnel: w195 -> [_ w205]
              tunnel: w194 -> [w199 w203]
              tunnel: [w199 w202] -> w193
              frame False {
              }
              frame True {
                w204 = u8 1 items=["1", "2", "3", "4", "5", "6", "7", "8", "9"] ("axis no")
                n109 = local read "axis 2:\nsp position °"() -> (w201:dbl)
                n110 = local read "axis 2:\nsp rot count"() -> (w200:i32)
                n111 = call "ANC350_MoveRelative.vi"("device handle"=w205, "axis no"=w204, "distance [µm/°/m°]"=w201, "rot count"=w200, "error in"=w203) -> ("error out"=w202:T6)  [unwired: 9 in, 1 out]
              }
            }
            n112 = call <vilib>:"Add State(s) to Queue__JKI_lib_State_Machine.vi"("State(s) in (\"\")"=w198) -> ("States Out"=w197:string)  [unwired: 14 in]
          }
          event "axis 1:\nsingle step fwd": Value Change {
            n113 = event-data() -> ()  [unwired: 1 in, 6 out]
            n114 = Unbundle By Name(w210) -> ("handle"=w209:i32)
            n115 = case shown="True" "axis 1:\nsingle step fwd" {
              tunnel: w209 -> [_ w218]
              tunnel: w208 -> [w213 w215]
              tunnel: [w213 w214] -> w207
              frame False {
              }
              frame True {
                w217 = u8 0 items=["1", "2", "3", "4", "5", "6", "7", "8", "9"] ("axis no")
                n116 = call "ANC350_MoveSingleStep.vi"("error in"=w215, "single step direction"=FALSE, "axis no"=w217, "device handle"=w218) -> ("error out"=w214:T6)  [unwired: 2 in, 1 out]
              }
            }
            n117 = call <vilib>:"Add State(s) to Queue__JKI_lib_State_Machine.vi"("State(s) in (\"\")"=w212) -> ("States Out"=w211:string)  [unwired: 14 in]
          }
          event "axis 1:\nsingle step back": Value Change {
            n118 = event-data() -> ()  [unwired: 1 in, 6 out]
            n119 = Unbundle By Name(w223) -> ("handle"=w222:i32)
            n120 = case shown="True" "axis 1:\nsingle step back" {
              tunnel: w222 -> [_ w231]
              tunnel: w221 -> [w226 w228]
              tunnel: [w226 w227] -> w220
              frame False {
              }
              frame True {
                w230 = u8 0 items=["1", "2", "3", "4", "5", "6", "7", "8", "9"] ("axis no")
                n121 = call "ANC350_MoveSingleStep.vi"("error in"=w228, "single step direction"=TRUE, "axis no"=w230, "device handle"=w231) -> ("error out"=w227:T6)  [unwired: 2 in, 1 out]
              }
            }
            n122 = call <vilib>:"Add State(s) to Queue__JKI_lib_State_Machine.vi"("State(s) in (\"\")"=w225) -> ("States Out"=w224:string)  [unwired: 14 in]
          }
          event "axis 2:\nsingle step fwd": Value Change {
            n123 = event-data() -> ()  [unwired: 1 in, 6 out]
            n124 = Unbundle By Name(w236) -> ("handle"=w235:i32)
            n125 = case shown="True" "axis 2:\nsingle step fwd" {
              tunnel: w235 -> [_ w244]
              tunnel: w234 -> [w239 w241]
              tunnel: [w239 w240] -> w233
              frame False {
              }
              frame True {
                w243 = u8 1 items=["1", "2", "3", "4", "5", "6", "7", "8", "9"] ("axis no")
                n126 = call "ANC350_MoveSingleStep.vi"("error in"=w241, "single step direction"=FALSE, "axis no"=w243, "device handle"=w244) -> ("error out"=w240:T6)  [unwired: 2 in, 1 out]
              }
            }
            n127 = call <vilib>:"Add State(s) to Queue__JKI_lib_State_Machine.vi"("State(s) in (\"\")"=w238) -> ("States Out"=w237:string)  [unwired: 14 in]
          }
          event "axis 2:\nsingle step back": Value Change {
            n128 = event-data() -> ()  [unwired: 1 in, 6 out]
            n129 = Unbundle By Name(w249) -> ("handle"=w248:i32)
            n130 = case shown="False" "axis 2:\nsingle step back" {
              tunnel: w248 -> [_ w257]
              tunnel: w247 -> [w252 w254]
              tunnel: [w252 w253] -> w246
              frame False {
              }
              frame True {
                w256 = u8 1 items=["1", "2", "3", "4", "5", "6", "7", "8", "9"] ("axis no")
                n131 = call "ANC350_MoveSingleStep.vi"("error in"=w254, "single step direction"=TRUE, "axis no"=w256, "device handle"=w257) -> ("error out"=w253:T6)  [unwired: 2 in, 1 out]
              }
            }
            n132 = call <vilib>:"Add State(s) to Queue__JKI_lib_State_Machine.vi"("State(s) in (\"\")"=w251) -> ("States Out"=w250:string)  [unwired: 14 in]
          }
          event "axis 1:\ncontinuous fwd": Value Change {
            n133 = event-data() -> ()  [unwired: 1 in, 6 out]
            n134 = Unbundle By Name(w262) -> ("handle"=w261:i32)
            n135 = case shown="False" "axis 1:\ncontinuous fwd" {
              tunnel: w261 -> [w268 w273]
              tunnel: w260 -> [w267 w271]
              tunnel: [w266 w270] -> w259
              frame False {
                w265 = u8 0 items=["1", "2", "3", "4", "5", "6", "7", "8", "9"] ("axis no")
                n136 = call "ANC350_StopMoving.vi"("error in"=w267, "axis no"=w265, "device handle"=w268) -> ("error out"=w266:T6)  [unwired: 3 in, 1 out]
              }
              frame True {
                w272 = u8 0 items=["1", "2", "3", "4", "5", "6", "7", "8", "9"] ("axis no")
                n137 = call "ANC350_MoveContinuous.vi"("error in"=w271, "step direction"=FALSE ("single step direction"), "axis no"=w272, "device handle"=w273) -> ("error out"=w270:T6)  [unwired: 2 in, 1 out]
              }
            }
            n138 = call <vilib>:"Add State(s) to Queue__JKI_lib_State_Machine.vi"("State(s) in (\"\")"=w264) -> ("States Out"=w263:string)  [unwired: 14 in]
          }
          event "axis 1:\ncontinuous back": Value Change {
            n139 = event-data() -> ()  [unwired: 1 in, 6 out]
            n140 = Unbundle By Name(w278) -> ("handle"=w277:i32)
            n141 = case shown="True" "axis 1:\ncontinuous back" {
              tunnel: w277 -> [w284 w289]
              tunnel: w276 -> [w283 w287]
              tunnel: [w282 w286] -> w275
              frame False {
                w281 = u8 0 items=["1", "2", "3", "4", "5", "6", "7", "8", "9"] ("axis no")
                n142 = call "ANC350_StopMoving.vi"("error in"=w283, "axis no"=w281, "device handle"=w284) -> ("error out"=w282:T6)  [unwired: 3 in, 1 out]
              }
              frame True {
                w288 = u8 0 items=["1", "2", "3", "4", "5", "6", "7", "8", "9"] ("axis no")
                n143 = call "ANC350_MoveContinuous.vi"("error in"=w287, "step direction"=TRUE ("single step direction"), "axis no"=w288, "device handle"=w289) -> ("error out"=w286:T6)  [unwired: 2 in, 1 out]
              }
            }
            n144 = call <vilib>:"Add State(s) to Queue__JKI_lib_State_Machine.vi"("State(s) in (\"\")"=w280) -> ("States Out"=w279:string)  [unwired: 14 in]
          }
          event "axis 2:\ncontinuous fwd": Value Change {
            n145 = event-data() -> ()  [unwired: 1 in, 6 out]
            n146 = Unbundle By Name(w294) -> ("handle"=w293:i32)
            n147 = case shown="False" "axis 2:\ncontinuous fwd" {
              tunnel: w293 -> [w300 w305]
              tunnel: w292 -> [w299 w303]
              tunnel: [w298 w302] -> w291
              frame False {
                w297 = u8 1 items=["1", "2", "3", "4", "5", "6", "7", "8", "9"] ("axis no")
                n148 = call "ANC350_StopMoving.vi"("error in"=w299, "axis no"=w297, "device handle"=w300) -> ("error out"=w298:T6)  [unwired: 3 in, 1 out]
              }
              frame True {
                w304 = u8 1 items=["1", "2", "3", "4", "5", "6", "7", "8", "9"] ("axis no")
                n149 = call "ANC350_MoveContinuous.vi"("error in"=w303, "step direction"=FALSE ("single step direction"), "axis no"=w304, "device handle"=w305) -> ("error out"=w302:T6)  [unwired: 2 in, 1 out]
              }
            }
            n150 = call <vilib>:"Add State(s) to Queue__JKI_lib_State_Machine.vi"("State(s) in (\"\")"=w296) -> ("States Out"=w295:string)  [unwired: 14 in]
          }
          event "axis 2:\ncontinuous back": Value Change {
            n151 = event-data() -> ()  [unwired: 1 in, 6 out]
            n152 = Unbundle By Name(w310) -> ("handle"=w309:i32)
            n153 = case shown="False" "axis 2:\ncontinuous back" {
              tunnel: w309 -> [w316 w321]
              tunnel: w308 -> [w315 w319]
              tunnel: [w314 w318] -> w307
              frame False {
                w313 = u8 1 items=["1", "2", "3", "4", "5", "6", "7", "8", "9"] ("axis no")
                n154 = call "ANC350_StopMoving.vi"("error in"=w315, "axis no"=w313, "device handle"=w316) -> ("error out"=w314:T6)  [unwired: 3 in, 1 out]
              }
              frame True {
                w320 = u8 1 items=["1", "2", "3", "4", "5", "6", "7", "8", "9"] ("axis no")
                n155 = call "ANC350_MoveContinuous.vi"("error in"=w319, "step direction"=TRUE ("single step direction"), "axis no"=w320, "device handle"=w321) -> ("error out"=w318:T6)  [unwired: 2 in, 1 out]
              }
            }
            n156 = call <vilib>:"Add State(s) to Queue__JKI_lib_State_Machine.vi"("State(s) in (\"\")"=w312) -> ("States Out"=w311:string)  [unwired: 14 in]
          }
          event "axis 1:\nAmplitude [V]": Value Change {
            w325 = u8 0 items=["1", "2", "3", "4", "5", "6", "7", "8", "9"] ("axis no")
            n157 = event-data() -> ()  [unwired: 1 in, 6 out]
            n158 = Unbundle By Name(w327) -> ("handle"=w326:i32)
            n159 = call "ANC350_Amplitude.vi"("error in"=w323, "PositionerAmplitude [V]"="axis 1:\nAmplitude [V]", "axis no"=w325, "device handle"=w326) -> ("error out"=w322:T6)  [unwired: 2 in, 1 out]
            n160 = call <vilib>:"Add State(s) to Queue__JKI_lib_State_Machine.vi"("State(s) in (\"\")"=w329) -> ("States Out"=w328:string)  [unwired: 14 in]
          }
          event "axis 2:\nAmplitude [V]": Value Change {
            w333 = u8 1 items=["1", "2", "3", "4", "5", "6", "7", "8", "9"] ("axis no")
            n161 = event-data() -> ()  [unwired: 1 in, 6 out]
            n162 = Unbundle By Name(w335) -> ("handle"=w334:i32)
            n163 = call "ANC350_Amplitude.vi"("error in"=w332, "PositionerAmplitude [V]"="axis 2:\nAmplitude [V]", "axis no"=w333, "device handle"=w334) -> ("error out"=w331:T6)  [unwired: 2 in, 1 out]
            n164 = call <vilib>:"Add State(s) to Queue__JKI_lib_State_Machine.vi"("State(s) in (\"\")"=w337) -> ("States Out"=w336:string)  [unwired: 14 in]
          }
          event "axis 1:\nDCLevel [V]": Value Change {
            w341 = u8 0 items=["1", "2", "3", "4", "5", "6", "7", "8", "9"] ("axis no")
            n165 = event-data() -> ()  [unwired: 1 in, 6 out]
            n166 = Unbundle By Name(w343) -> ("handle"=w342:i32)
            n167 = call "ANC350_DCLevel.vi"("error in"=w339, "DCLevel [V]"="axis 1:\nDCLevel [V]", "axis no"=w341, "device handle"=w342) -> ("error out"=w338:T6)  [unwired: 2 in, 1 out]
            n168 = call <vilib>:"Add State(s) to Queue__JKI_lib_State_Machine.vi"("State(s) in (\"\")"=w345) -> ("States Out"=w344:string)  [unwired: 14 in]
          }
          event "axis 2:\nDCLevel [V]": Value Change {
            w349 = u8 1 items=["1", "2", "3", "4", "5", "6", "7", "8", "9"] ("axis no")
            n169 = event-data() -> ()  [unwired: 1 in, 6 out]
            n170 = Unbundle By Name(w351) -> ("handle"=w350:i32)
            n171 = call "ANC350_DCLevel.vi"("error in"=w348, "DCLevel [V]"="axis 2:\nDCLevel [V]", "axis no"=w349, "device handle"=w350) -> ("error out"=w347:T6)  [unwired: 2 in, 1 out]
            n172 = call <vilib>:"Add State(s) to Queue__JKI_lib_State_Machine.vi"("State(s) in (\"\")"=w353) -> ("States Out"=w352:string)  [unwired: 14 in]
          }
          event "axis 1:\nFrequency [Hz]": Value Change {
            w357 = u8 0 items=["1", "2", "3", "4", "5", "6", "7", "8", "9"] ("axis no")
            n173 = event-data() -> ()  [unwired: 1 in, 6 out]
            n174 = Unbundle By Name(w359) -> ("handle"=w358:i32)
            n175 = call "ANC350_Frequency.vi"("error in"=w355, "PositionerFrequency [Hz]"="axis 1:\nFrequency [Hz]", "axis no"=w357, "device handle"=w358) -> ("error out"=w354:T6)  [unwired: 2 in, 1 out]
            n176 = call <vilib>:"Add State(s) to Queue__JKI_lib_State_Machine.vi"("State(s) in (\"\")"=w361) -> ("States Out"=w360:string)  [unwired: 14 in]
          }
          event "axis 2:\nFrequency [Hz]": Value Change {
            w365 = u8 1 items=["1", "2", "3", "4", "5", "6", "7", "8", "9"] ("axis no")
            n177 = event-data() -> ()  [unwired: 1 in, 6 out]
            n178 = Unbundle By Name(w367) -> ("handle"=w366:i32)
            n179 = call "ANC350_Frequency.vi"("error in"=w364, "PositionerFrequency [Hz]"="axis 2:\nFrequency [Hz]", "axis no"=w365, "device handle"=w366) -> ("error out"=w363:T6)  [unwired: 2 in, 1 out]
            n180 = call <vilib>:"Add State(s) to Queue__JKI_lib_State_Machine.vi"("State(s) in (\"\")"=w369) -> ("States Out"=w368:string)  [unwired: 14 in]
          }
          event "axis 1:\ncap. measure": Value Change {
            w373 = u8 0 items=["1", "2", "3", "4", "5", "6", "7", "8", "9"] ("axis no")
            n181 = event-data() -> ()  [unwired: 1 in, 6 out]
            n182 = Unbundle By Name(w375) -> ("handle"=w374:i32)
            n183 = case shown="True" "axis 1:\ncap. measure" {
              tunnel: w374 -> [_ w383]
              tunnel: w373 -> [_ w382]
              tunnel: w372 -> [w378 w381]
              tunnel: [w378 w380] -> w371
              frame False {
              }
              frame True {
                n184 = call "ANC350_CapMeasure.vi"("error in"=w381, "axis no"=w382, "device handle"=w383) -> ("error out"=w380:T6, "Capacitance"=→"axis 1:\nCapacitance":i32)  [unwired: 2 in, 1 out]
              }
            }
            n185 = call <vilib>:"Add State(s) to Queue__JKI_lib_State_Machine.vi"("State(s) in (\"\")"=w377) -> ("States Out"=w376:string)  [unwired: 14 in]
          }
          event "axis 2:\ncap. measure": Value Change {
            w387 = u8 1 items=["1", "2", "3", "4", "5", "6", "7", "8", "9"] ("axis no")
            n186 = event-data() -> ()  [unwired: 1 in, 6 out]
            n187 = Unbundle By Name(w389) -> ("handle"=w388:i32)
            n188 = case shown="True" "axis 2:\ncap. measure" {
              tunnel: w388 -> [_ w397]
              tunnel: w387 -> [_ w396]
              tunnel: w386 -> [w392 w395]
              tunnel: [w392 w394] -> w385
              frame False {
              }
              frame True {
                n189 = call "ANC350_CapMeasure.vi"("error in"=w395, "axis no"=w396, "device handle"=w397) -> ("error out"=w394:T6, "Capacitance"=→"axis 2:\nCapacitance":i32)  [unwired: 2 in, 1 out]
              }
            }
            n190 = call <vilib>:"Add State(s) to Queue__JKI_lib_State_Machine.vi"("State(s) in (\"\")"=w391) -> ("States Out"=w390:string)  [unwired: 14 in]
          }
          event "axis 1:\ncontrol mode": Value Change {
            w401 = u8 0 items=["1", "2", "3", "4", "5", "6", "7", "8", "9"] ("axis no")
            n191 = event-data() -> ()  [unwired: 1 in, 6 out]
            n192 = Unbundle By Name(w403) -> ("handle"=w402:i32)
            n193 = call "ANC350_AmplitudeControl.vi"("error in"=w400, "control mode"="axis 1:\ncontrol mode", "axis no"=w401, "device handle"=w402) -> ("error out"=w399:T6)  [unwired: 2 in, 1 out]
            n194 = call <vilib>:"Add State(s) to Queue__JKI_lib_State_Machine.vi"("State(s) in (\"\")"=w405) -> ("States Out"=w404:string)  [unwired: 14 in]
          }
          event "axis 2:\ncontrol mode": Value Change {
            w409 = u8 1 items=["1", "2", "3", "4", "5", "6", "7", "8", "9"] ("axis no")
            n195 = event-data() -> ()  [unwired: 1 in, 6 out]
            n196 = Unbundle By Name(w411) -> ("handle"=w410:i32)
            n197 = call "ANC350_AmplitudeControl.vi"("error in"=w408, "control mode"="axis 2:\ncontrol mode", "axis no"=w409, "device handle"=w410) -> ("error out"=w407:T6)  [unwired: 2 in, 1 out]
            n198 = call <vilib>:"Add State(s) to Queue__JKI_lib_State_Machine.vi"("State(s) in (\"\")"=w413) -> ("States Out"=w412:string)  [unwired: 14 in]
          }
          event "axis 1:\nOutput": Value Change {
            w415 = u8 0 items=["1", "2", "3", "4", "5", "6", "7", "8", "9"] ("axis no")
            n199 = event-data() -> ()  [unwired: 1 in, 6 out]
            n200 = Unbundle By Name(w419) -> ("handle"=w418:i32)
            n201 = call "ANC350_SetOutput.vi"("error in"=w417, "enable"="axis 1:\nOutput", "axis no"=w415, "device handle"=w418) -> ("error out"=w416:T6)  [unwired: 2 in, 1 out]
            n202 = call <vilib>:"Add State(s) to Queue__JKI_lib_State_Machine.vi"("State(s) in (\"\")"=w421) -> ("States Out"=w420:string)  [unwired: 14 in]
          }
          event "axis 2:\nOutput": Value Change {
            w423 = u8 1 items=["1", "2", "3", "4", "5", "6", "7", "8", "9"] ("axis no")
            n203 = event-data() -> ()  [unwired: 1 in, 6 out]
            n204 = Unbundle By Name(w427) -> ("handle"=w426:i32)
            n205 = call "ANC350_SetOutput.vi"("error in"=w425, "enable"="axis 2:\nOutput", "axis no"=w423, "device handle"=w426) -> ("error out"=w424:T6)  [unwired: 2 in, 1 out]
            n206 = call <vilib>:"Add State(s) to Queue__JKI_lib_State_Machine.vi"("State(s) in (\"\")"=w429) -> ("States Out"=w428:string)  [unwired: 14 in]
          }
          event "axis 1:\nstop detection": Value Change {
            w433 = u8 0 items=["1", "2", "3", "4", "5", "6", "7", "8", "9"] ("axis no")
            n207 = event-data() -> ()  [unwired: 1 in, 6 out]
            n208 = Unbundle By Name(w435) -> ("handle"=w434:i32)
            n209 = call "ANC350_StopDetection.vi"("error in"=w432, "enable"="axis 1:\nstop detection", "axis no"=w433, "device handle"=w434) -> ("error out"=w431:T6)  [unwired: 2 in, 1 out]
            n210 = call <vilib>:"Add State(s) to Queue__JKI_lib_State_Machine.vi"("State(s) in (\"\")"=w437) -> ("States Out"=w436:string)  [unwired: 14 in]
          }
          event "axis 2:\nstop detection": Value Change {
            w441 = u8 1 items=["1", "2", "3", "4", "5", "6", "7", "8", "9"] ("axis no")
            n211 = event-data() -> ()  [unwired: 1 in, 6 out]
            n212 = Unbundle By Name(w443) -> ("handle"=w442:i32)
            n213 = call "ANC350_StopDetection.vi"("error in"=w440, "enable"="axis 2:\nstop detection", "axis no"=w441, "device handle"=w442) -> ("error out"=w439:T6)  [unwired: 2 in, 1 out]
            n214 = call <vilib>:"Add State(s) to Queue__JKI_lib_State_Machine.vi"("State(s) in (\"\")"=w445) -> ("States Out"=w444:string)  [unwired: 14 in]
          }
          event "axis 1:\nStop moving": Value Change {
            w449 = u8 0 items=["1", "2", "3", "4", "5", "6", "7", "8", "9"] ("axis no")
            n215 = event-data() -> ()  [unwired: 1 in, 6 out]
            n216 = Unbundle By Name(w451) -> ("handle"=w450:i32)
            n217 = case shown="False" "axis 1:\nStop moving" {
              tunnel: w450 -> [_ w458]
              tunnel: w449 -> [_ w457]
              tunnel: w448 -> [w454 w456]
              tunnel: [w454 w455] -> w447
              frame False {
              }
              frame True {
                n218 = call "ANC350_StopMoving.vi"("error in"=w456, "axis no"=w457, "device handle"=w458) -> ("error out"=w455:T6)  [unwired: 3 in, 1 out]
              }
            }
            n219 = call <vilib>:"Add State(s) to Queue__JKI_lib_State_Machine.vi"("State(s) in (\"\")"=w453) -> ("States Out"=w452:string)  [unwired: 14 in]
          }
          event "axis 2:\nStop moving": Value Change {
            w462 = u8 1 items=["1", "2", "3", "4", "5", "6", "7", "8", "9"] ("axis no")
            n220 = event-data() -> ()  [unwired: 1 in, 6 out]
            n221 = Unbundle By Name(w464) -> ("handle"=w463:i32)
            n222 = case shown="True" "axis 2:\nStop moving" {
              tunnel: w463 -> [_ w471]
              tunnel: w462 -> [_ w470]
              tunnel: w461 -> [w467 w469]
              tunnel: [w467 w468] -> w460
              frame False {
              }
              frame True {
                n223 = call "ANC350_StopMoving.vi"("error in"=w469, "axis no"=w470, "device handle"=w471) -> ("error out"=w468:T6)  [unwired: 3 in, 1 out]
              }
            }
            n224 = call <vilib>:"Add State(s) to Queue__JKI_lib_State_Machine.vi"("State(s) in (\"\")"=w466) -> ("States Out"=w465:string)  [unwired: 14 in]
          }
          event "both axes: Output": Value Change {
            n225 = event-data() -> ()  [unwired: 1 in, 6 out]
            n226 = local write "axis 2:\nOutput"("both axes: Output") -> ()
            n227 = local write "axis 1:\nOutput"("both axes: Output") -> ()
            n228 = property on="axis 1:\nOutput" class="Bool (strict)"("Val(Sgnl)"="both axes: Output") -> ()  [unwired: 2 in, 2 out]
            n229 = property on="axis 2:\nOutput" class="Bool (strict)"("Val(Sgnl)"="both axes: Output") -> ()  [unwired: 2 in, 2 out]
            n230 = call <vilib>:"Add State(s) to Queue__JKI_lib_State_Machine.vi"("State(s) in (\"\")"=w476) -> ("States Out"=w475:string)  [unwired: 14 in]
          }
          event "static amplitude (mV)": Value Change {
            n231 = event-data() -> ()  [unwired: 1 in, 6 out]
            n232 = local read "set static amplitude\nwhen moving"() -> (w477:bool)
            n233 = local read "static amplitude (mV)"() -> (w478:dbl)
            n234 = Unbundle By Name(w482) -> ("handle"=w481:i32)
            n235 = case shown="False" w477 {
              tunnel: w481 -> [w488 _]
              tunnel: w480 -> [w487 w489]
              tunnel: [w486 w489] -> w479
              tunnel: w478 -> [w485 _]
              frame False {
                n236 = call "ANC350_StaticAmplitude.vi"("error in"=w487, "static amplitude"=w485, "device handle"=w488) -> ("error out"=w486:T6)  [unwired: 3 in, 1 out]
              }
              frame True {
              }
            }
            n237 = call <vilib>:"Add State(s) to Queue__JKI_lib_State_Machine.vi"("State(s) in (\"\")"=w484) -> ("States Out"=w483:string)  [unwired: 14 in]
          }
          event Panel Close? {
            # "Discard the event because we'll close the front panel ourselves in Macro: Exit"
            # "Close Panel button (pressed) Event\n(this executes Macro: Exit to terminate the VI)"
            n238 = event-data() -> ()  [unwired: 1 in, 1 out]
            n239 = call <vilib>:"Add State(s) to Queue__JKI_lib_State_Machine.vi"("State(s) in Front (\"\")"="Macro: Exit", "State(s) in (\"\")"=w495) -> ("States Out"=w494:string)  [unwired: 13 in]
            n240 = event-data("Discard?"=TRUE) -> ()  [unwired: 1 in, 1 out]
          }
        }
      }
      frame "---------- Core ----------" {
        # "Do not put any code in this frame.\n(it is a separator no-op)"
        n241 = call <vilib>:"Add State(s) to Queue__JKI_lib_State_Machine.vi"("State(s) in (\"\")"=w499) -> ("States Out"=w498:string)  [unwired: 14 in]
      }
      frame Default {
        w509 = 42 items=["No error", "Argument error", "Memory is full", "Out of zone", "End of file", "File already open", "Generic file I/O error", "File not found", "File permission error", "Disk is full", "Duplicate path", "Too many files open", "System feature not enabled", "Resource file not found", "Cannot add resource", "Resource not found", "Image not found", "Image memory error", "Pen does not exist", "Config type invalid", "Config token not found", "Config parse error", "Config memory error", "Bad external code format", "Bad external code offset", "External code not present", "Null window", "Destroy window error", "Null menu", "Print aborted", "Bad print record", "Print driver error", "Windows error during printing", "Memory error during printing", "Print dialog error", "Generic print error", "Invalid device refnum", "Device not found", "Device parameter error", "Device unit error", "Cannot open device", "Device call aborted", "Generic error", "Cancelled by user", "Object ID too low", "Object ID too high", "Object not in heap", "Unknown heap", "Unknown object (invalid DefProc)", "Unknown object (DefProc not in table)", "Message out of range", "Invalid (null) method", "Unknown message", "Manager call not supported", "Bad address", "Network operation in progress", "Network operation timed out", "Connection is busy", "Network attribute not supported", "Network error", "Address in use", "System out of memory", "Connection aborted", "Connection refused", "Not connected", "Already connected", "Connection closed", "Initialization error (interapplication manager)", "Bad occurrence", "Wait on unbound occurrence handler", "Occurrence queue overflow", "Datalog type conflict", "Unused", "Unrecognized type (interapplication manager)", "Memory corrupt", "Failed to make temporary DLL", "Old CIN version", "Drag socket not found", "Failed to load drop-object", "Failed to register OLE object", "Failed to release OLE object", "Format specifier type mismatch", "Unknown format specifier", "Too few format specifiers", "Too many format specifiers", "Scan failed", "Newer CIN version", "Error converting to variant", "Runtime menu error", "Password tampered", "Variant attribute not found", "Incompatible variant data type", "Event data is not available", "Event Store is not present", "Occurrence is not found", "Event Queue is not created", "Event info is not available", "Refnum passed is NULL", "Error retrieving Class GUID", "Error retrieving CoClass GUID", "Error retrieving TypeLib GUID.", "Bad built application magic bytes.", "Specific driver is different from the specific driver associated with the Logical Name.", "There is no session opened to the class driver.", "Max Error", "MAX - Error with config objects", "MAX - Error loading configuration", "MAX - Group not supported"]
        # "Current State"
        # "Do not delete, rename, or modify this frame.\n(this is used to capture unhandled states and typos)"
        # "Handle mistyped state name (developer tool)"
        n242 = Format Into String(format string="Software Exception: Unhandled State \"%s\"." ("message"), error in=w505, w500) -> (resulting string=w508:string, error out=w507:errorcluster)  [unwired: 1 in]
        n243 = call <vilib>:"Error Cluster From Error Code.vi"("show call chain? (False)"=TRUE, "error in (no error)"=w507, "error message (\"\")"=w508, "error code (0)"=w509) -> ("error out"=w506:errorcluster)  [unwired: 5 in]
        n244 = call <vilib>:"Add State(s) to Queue__JKI_lib_State_Machine.vi"("State(s) in (\"\")"=w504) -> ("States Out"=w503:string)  [unwired: 14 in]
      }
      frame "Initialize Core Data" {
        # "Do not delete, rename, or modify this frame.\n(this is used to determine panel behavior on exit)"
        # "originally closed?"
        # "exe?"
        # "If panel starts closed or is an EXE, then close it when we exit"
        n245 = property class="VI"() -> ("Front Panel.Open"=w518:bool)  [unwired: 2 in, 2 out]
        n246 = property class="App"() -> ("App.Kind"=w517:T2)  [unwired: 2 in, 2 out]
        n247 = control-ref of="Current VI Reference"() -> (w511:refnum<vi>)
        n248 = Not(x=w518) -> (.not. x?=w515:bool)
        n249 = Equal?(x=w517, y=T2."Run Time System" ("Application:Kind")) -> (x = y?=w514:bool)
        n250 = Or(x=w515, y=w514) -> (x .or. y?=w512:bool)
        n251 = Bundle By Name(cluster=w513, "Core.Current VI Reference"=w511, "Core.Close Panel on Exit?"=w512) -> (w520:T7)
        n252 = call <vilib>:"Add State(s) to Queue__JKI_lib_State_Machine.vi"("State(s) in (\"\")"=w522) -> ("States Out"=w521:string)  [unwired: 14 in]
      }
      frame "Error Handler" {
        # "Unhandled Error -- Display it"
        # "Handle any errors here.\nYou can also output any states to clean-up after errors occur"
        # "Clear error"
        n253 = call <vilib>:"General Error Handler.vi"("error in (no error)"=w524) -> ()  [unwired: 10 in, 5 out]
        n254 = call <vilib>:"Add State(s) to Queue__JKI_lib_State_Machine.vi"("State(s) in Front (\"\")"="/* Post Error States", "State(s) in (\"\")"=w528) -> ("States Out"=w527:string)  [unwired: 13 in]
      }
      frame "Exit" {
        # "Do not put any code in this frame.\n(No errors that occur here will be handled.)"
        n255 = call <vilib>:"Add State(s) to Queue__JKI_lib_State_Machine.vi"("State(s) in (\"\")"=w533) -> ("States Out"=w532:string)  [unwired: 14 in]
      }
      frame "---------- Data ----------" {
        # "Do not put any code in this frame.\n(It is a separator no-op. You can make a copy of this frame to create a new Data frame)"
        n256 = call <vilib>:"Add State(s) to Queue__JKI_lib_State_Machine.vi"("State(s) in (\"\")"=w537) -> ("States Out"=w536:string)  [unwired: 14 in]
      }
      frame "Data: Initialize" {
        w538 = 0  # handle
        w539 = T8 {"Current VI Reference"=refnum, "Close Panel on Exit?"=FALSE}  # Core
        # "do not delete - used by framework"
        # "Expand Bundle to add new data elements to shift register data."
        # "Data names and types of shift register data are defined by this bundle."
        # "Initialize the shift-register data, here.\n(data names are defined by what you wire into the bundle function)"
        n257 = Bundle("Core"=w539, "handle"=w538) -> (w541:T7)  [unwired: 1 in]
        n258 = call <vilib>:"Add State(s) to Queue__JKI_lib_State_Machine.vi"("State(s) in (\"\")"=w543) -> ("States Out"=w542:string)  [unwired: 14 in]
      }
      frame "Data: Cleanup" {
        # "Cleanup any data and references, here.\n(this is called automatically, by the Macro: Exit)"
        n259 = Unbundle By Name(w544) -> ("Core.Current VI Reference"=w547:refnum<vi>)
        n260 = Close Reference(reference=w547, error in (no error)=w546) -> (error out=w545:errorcluster)
        n261 = call <vilib>:"Add State(s) to Queue__JKI_lib_State_Machine.vi"("State(s) in (\"\")"=w549) -> ("States Out"=w548:string)  [unwired: 14 in]
      }
      frame "---------- UI ----------" {
        # "Do not put any code in this frame.\n(It is a separator no-op. You can make a copy of this frame to create a new UI frame)"
        n262 = call <vilib>:"Add State(s) to Queue__JKI_lib_State_Machine.vi"("State(s) in (\"\")"=w553) -> ("States Out"=w552:string)  [unwired: 14 in]
      }
      frame "UI: Initialize" {
        w554 = FALSE ("OK")
        w558 = FALSE ("axis 1:\nAbsolute")
        w559 = FALSE ("axis 1:\nAbsolute")
        w556 = FALSE ("axis 1:\nAbsolute")
        w560 = FALSE ("axis 1: \nTarget GND")
        # "initialize buttons and graphs....."
        # "Initialize the User Interface, here.\n(this is called automatically, by the Macro: Init)"
        n263 = local write "axis 1:\nSingle Circle Mode"(TRUE ("axis 1: \nTarget GND")) -> ()
        n264 = local write "axis 2:\nSingle Circle Mode"(FALSE ("axis 1:\nAbsolute")) -> ()
        n265 = local write "axis 1: \nTarget GND"(w560) -> ()
        n266 = local write "axis 2: \nTarget GND"(w560) -> ()
        n267 = local write "axis 2:\nAbsolute"(w556) -> ()
        n268 = local write "axis 1:\nAbsolute"(w556) -> ()
        n269 = local write "axis 1:\nRelative"(w556) -> ()
        n270 = local write "axis 2:\nRelative"(w556) -> ()
        n271 = local write "axis 2:\ncap. measure"(w558) -> ()
        n272 = local write "axis 1:\ncap. measure"(w558) -> ()
        n273 = local write "axis 2:\nOutput"(w556) -> ()
        n274 = local write "axis 1:\nOutput"(w556) -> ()
        n275 = local write "axis 1:\nsingle step back"(w559) -> ()
        n276 = local write "axis 1:\nsingle step fwd"(w559) -> ()
        n277 = local write "axis 2:\nsingle step back"(w559) -> ()
        n278 = local write "axis 2:\nsingle step fwd"(w559) -> ()
        n279 = local write "axis 1:\ncontinuous back"(w559) -> ()
        n280 = local write "axis 1:\ncontinuous fwd"(w559) -> ()
        n281 = local write "axis 2:\ncontinuous back"(w559) -> ()
        n282 = local write "axis 2:\ncontinuous fwd"(w559) -> ()
        n283 = local write "OK"(w554) -> ()
        n284 = local write "Remote mode"(w554) -> ()
        n285 = local write "both axes: Output"(w554) -> ()
        n286 = disable-structure shown="Disabled" {
          frame Disabled {
            w565 = 0.0 ("axis 1:\nAmplitude [V]")
            w566 = 0 ("axis 1:\nFrequency [Hz]")
            w567 = 0.0 ("axis 1:\nAmplitude [V]")
            w568 = 1000 ("axis 1:\nFrequency [Hz]")
            w569 = 30.0 ("axis 1:\nAmplitude [V]")
            n287 = local write "axis 1:\nAmplitude [V]"(w569) -> ()
            n288 = local write "axis 2:\nAmplitude [V]"(w569) -> ()
            n289 = local write "axis 1:\nFrequency [Hz]"(w568) -> ()
            n290 = local write "axis 2:\nFrequency [Hz]"(w568) -> ()
            n291 = local write "axis 1:\nDCLevel [V]"(w567) -> ()
            n292 = local write "axis 1:\nsp rot count"(w566) -> ()
            n293 = local write "axis 2:\nDCLevel [V]"(w567) -> ()
            n294 = local write "axis 2:\nsp rot count"(w566) -> ()
            n295 = local write "axis 1:\nsp position °"(w565) -> ()
            n296 = local write "axis 2:\nsp position °"(w565) -> ()
          }
          frame Enabled {
          }
        }
        n297 = call <vilib>:"Add State(s) to Queue__JKI_lib_State_Machine.vi"("State(s) in (\"\")"=w564) -> ("States Out"=w563:string)  [unwired: 14 in]
      }
      frame "UI: Cursor Set" {
        # "Argument"
        # "Set and Unset Cursor Busy.\n(Usage: \"UI: Cursor Set >> Busy|Idle\")"
        n298 = case shown="\"Idle\", Default" w570 {
          tunnel: w572 -> [w577 w579]
          tunnel: [w576 w578] -> w571
          frame "Idle", Default {
            n299 = call <vilib>:"Unset Busy.vi"("error in (no error)"=w577) -> ("error out"=w576:errorcluster)  [unwired: 10 in]
          }
          frame "Busy" {
            n300 = call <vilib>:"Set Busy.vi"("error in (no error)"=w579) -> ("error out"=w578:errorcluster)  [unwired: 9 in, 1 out]
          }
        }
        n301 = call <vilib>:"Add State(s) to Queue__JKI_lib_State_Machine.vi"("State(s) in (\"\")"=w575) -> ("States Out"=w574:string)  [unwired: 14 in]
      }
      frame "UI: Front Panel State" {
        # "Argument"
        # "Set Front Panel Open or Closed\n(Usage: \"UI: Front Panel State >> Open|Close\")"
        n302 = Unbundle By Name(w582) -> ("Core.Current VI Reference"=w581:refnum<vi>)
        n303 = case shown="\"Open\", Default" w580 {
          tunnel: w584 -> [w590 w603]
          tunnel: [w592 w604] -> w583
          tunnel: w581 -> [w591 w601]
          frame "Open", Default {
            n304 = property class="VI"(reference=w591, error in=w590) -> (reference out=w588:refnum<vi>, error out=w589:errorcluster, "Front Panel.Open"=w587:bool)
            n305 = case shown="False" w587 {
              tunnel: [w595 w598] -> w592
              tunnel: w589 -> [w594 w598]
              tunnel: w588 -> [w593 _]
              frame False {
                n306 = invoke class="VI" method="FP.Open"(reference=w593, error in=w594, "Activate"=TRUE, "State"=T3."Standard") -> (error out=w595:errorcluster)  [unwired: 1 in, 4 out]
              }
              frame True {
              }
            }
          }
          frame "Close" {
            n307 = property class="VI"(reference=w601, error in=w603) -> (reference out=w600:refnum<vi>, error out=w602:errorcluster, "Front Panel.Open"=w599:bool)
            n308 = case shown="True" w599 {
              tunnel: [w605 w608] -> w604
              tunnel: w602 -> [w605 w607]
              tunnel: w600 -> [_ w606]
              frame False {
              }
              frame True {
                n309 = invoke class="VI" method="FP.Close"(reference=w606, error in=w607) -> (error out=w608:errorcluster)  [unwired: 1 in, 2 out]
              }
            }
          }
        }
        n310 = call <vilib>:"Add State(s) to Queue__JKI_lib_State_Machine.vi"("State(s) in (\"\")"=w586) -> ("States Out"=w585:string)  [unwired: 14 in]
      }
      frame "---------- Macro ----------" {
        # "Do not put any code in this frame.\n(It is a separator no-op. You can make a copy of this frame to create a new Macro frame)"
        n311 = call <vilib>:"Add State(s) to Queue__JKI_lib_State_Machine.vi"("State(s) in (\"\")"=w612) -> ("States Out"=w611:string)  [unwired: 14 in]
      }
      frame "Macro: Initialize" {
        w613 = "Data: Initialize\nInitialize Core Data\nUI: Initialize\nUI: Front Panel State >> Open\nAttocube: Initialize"  # Data: Initialize Initialize Core Data UI: Initialize UI: Front Panel State >> Open Attocube: Initialize
        # "Initialization Macro\n(This is called once, when the VI starts)"
        n312 = call <vilib>:"Add State(s) to Queue__JKI_lib_State_Machine.vi"("State(s) in Front (\"\")"=w613, "State(s) in (\"\")"=w617) -> ("States Out"=w616:string)  [unwired: 13 in]
      }
      frame "Macro: Exit" {
        w621 = u8 1 items=["1", "2", "3", "4", "5", "6", "7", "8", "9"] ("axis no")
        w624 = u8 0 items=["1", "2", "3", "4", "5", "6", "7", "8", "9"] ("axis no")
        w628 = u8 1 items=["1", "2", "3", "4", "5", "6", "7", "8", "9"] ("axis no")
        w629 = u8 0 items=["1", "2", "3", "4", "5", "6", "7", "8", "9"] ("axis no")
        # "Exit Macro\n(This is called once, when the VI exits)"
        n313 = Unbundle By Name(w641) -> ("Core.Close Panel on Exit?"=w640:bool, "handle"=w633:i32)
        n314 = call "ANC350_StopMoving.vi"("error in"=w631, "axis no"=w629, "device handle"=w633) -> ("error out"=w630:T6, "device handle Out"=w632:i32)  [unwired: 3 in]
        n315 = call "ANC350_StopMoving.vi"("error in"=w630, "axis no"=w628, "device handle"=w632) -> ("error out"=w625:T6, "device handle Out"=w627:i32)  [unwired: 3 in]
        n316 = call "ANC350_SetOutput.vi"("error in"=w625, "enable"=FALSE, "axis no"=w624, "device handle"=w627) -> ("error out"=w620:T6, "device handle out"=w623:i32)  [unwired: 2 in]
        n317 = Select(t="UI: Front Panel State >> Close", s=w640, f="") -> (s? t:f=w637:string)
        n318 = call "ANC350_SetOutput.vi"("error in"=w620, "enable"=FALSE, "axis no"=w621, "device handle"=w623) -> ("error out"=w618:T6, "device handle out"=w619:i32)  [unwired: 2 in]
        n319 = call <vilib>:"Add State(s) to Queue__JKI_lib_State_Machine.vi"("State(s) in (\"\")"=w637, "State(s) at Back (\"\")"="Data: Cleanup\nExit") -> ("States Out"=w635:string)  [unwired: 13 in]
        n320 = call "ANC350_Close.vi"("error in"=w618, "device handle"=w619) -> ("error out"=w634:T6)  [unwired: 5 in]
        n321 = call <vilib>:"Add State(s) to Queue__JKI_lib_State_Machine.vi"("State(s) in Front (\"\")"=w635, "State(s) in (\"\")"=w643) -> ("States Out"=w642:string)  [unwired: 13 in]
      }
      frame "---------- New Category ----------" {
        # "Template Separator\n(You can make a copy of, or modify, this frame)"
        n322 = call <vilib>:"Add State(s) to Queue__JKI_lib_State_Machine.vi"("State(s) in (\"\")"=w647) -> ("States Out"=w646:string)  [unwired: 14 in]
      }
      frame "Attocube: Initialize" {
        n323 = flat-sequence {
          tunnel: [w657] -> w650
          tunnel: [w656] -> w649
          frame #0 {
            n324 = call "ANC350_Check.vi"() -> ()  [unwired: 6 in, 2 out]
          }
          frame #1 {
            n325 = call "ANC350_Connect.vi"("device no"=0) -> ("error out"=w656:T6, "handle"=w657:i32)  [unwired: 5 in]
            "handle" <- w657
          }
        }
        n326 = Bundle By Name(cluster=w653, "handle"=w650) -> (w652:T7)
        n327 = Get Date/Time In Seconds() -> (seconds since 1Jan1904=w648:timestamp)
        n328 = local write "last move time"(w648) -> ()
        n329 = call <vilib>:"Add State(s) to Queue__JKI_lib_State_Machine.vi"("State(s) in (\"\")"=w655, "State(s) at Back (\"\")"="Attocube: Query\nAttocube: Log to DSC\nAttocube: FGV" ("State(s) at Back (\"\")")) -> ("States Out"=w654:string)  [unwired: 13 in]
      }
      frame "Attocube: Query" {
        w695 = u8 0 items=["1", "2", "3", "4", "5", "6", "7", "8", "9"] ("axis no")
        w702 = u8 1 items=["1", "2", "3", "4", "5", "6", "7", "8", "9"] ("axis no")
        w682 = u8 1 items=["1", "2", "3", "4", "5", "6", "7", "8", "9"] ("axis no")
        w703 = u8 0 items=["1", "2", "3", "4", "5", "6", "7", "8", "9"] ("axis no")
        w715 = u8 1 items=["1", "2", "3", "4", "5", "6", "7", "8", "9"] ("axis no")
        w717 = u8 0 items=["1", "2", "3", "4", "5", "6", "7", "8", "9"] ("axis no")
        n330 = Unbundle By Name(w719) -> ("handle"=w716:i32)
        n331 = local read "set static amplitude\nwhen moving"() -> (w659:bool)
        n332 = call "ANC350_GetRotCount.vi"("error in"=w718, "axis no"=w717, "device handle"=w716) -> ("error out"=w694:T6, "count"=→"axis 1:\nrot. count":i32, "device handle"=w696:i32)  [unwired: 2 in]
        n333 = call "ANC350_GetStatus.vi"("error in"=w694, "axis no"=w695, "device handle"=w696) -> ("error out"=w689:T6, "positioner status"=w687:T1, "axis no out"=w691:u8, "device handle Out"=w693:i32)  [unwired: 2 in, 3 out]
        "axis 1:\npositioner status" <- w687
        n334 = Unbundle By Name(w687) -> ("moving"=w663:bool)
        n335 = local read "axis 2:\nCurrent position (°)"() -> (w671:dbl)
        n336 = local read "axis 1:\nCurrent position (°)"() -> (w686:dbl)
        n337 = Not(x=w663) -> (.not. x?=w660:bool)
        n338 = call "ANC350_GetPosition.vi"("error in"=w689, "axis no"=w691, "device handle"=w693) -> ("error out"=w688:T6, "position [µm/°/m°]"=w685:dbl, "axis no out"=w690:u8, "device handle Out"=w692:i32)  [unwired: 1 in]
        n339 = And(x=w660, y=w659) -> (x .and. y?=w666:bool)
        n340 = Select(t=w686, s=w666, f=w685) -> (s? t:f=→"axis 1:\nCurrent position (°)" →"axis 1:\nCurrent position [µm/°/m°] 2":dbl)
        n341 = call "ANC350_GetSpeed.vi"("error in"=w688, "axis no"=w690, "device handle"=w692) -> ("error out"=w713:T6, "speed"=w707:i32, "device handle"=w714:i32)  [unwired: 2 in]
        n342 = call "ANC350_GetStepWidth.vi"("error in"=w713, "axis no"=w703, "device handle"=w714) -> ("error out"=w712:T6, "StepWidth"=→"axis 1:\nStepWidth":i32, "device handle"=w711:i32)  [unwired: 2 in]
        n343 = call "ANC350_GetRotCount.vi"("error in"=w712, "axis no"=w715, "device handle"=w711) -> ("error out"=w681:T6, "count"=→"axis 2:\nrot. count":i32, "device handle"=w683:i32)  [unwired: 2 in]
        n344 = call "ANC350_GetStatus.vi"("error in"=w681, "axis no"=w682, "device handle"=w683) -> ("error out"=w678:T6, "positioner status"=w674:T1, "axis no out"=w679:u8, "device handle Out"=w680:i32)  [unwired: 2 in, 3 out]
        "axis 2:\npositioner status" <- w674
        n345 = Unbundle By Name(w674) -> ("moving"=w662:bool)
        n346 = call "ANC350_GetPosition.vi"("error in"=w678, "axis no"=w679, "device handle"=w680) -> ("error out"=w677:T6, "position [µm/°/m°]"=w672:dbl, "axis no out"=w675:u8, "device handle Out"=w676:i32)  [unwired: 1 in]
        n347 = Not(x=w662) -> (.not. x?=w673:bool)
        n348 = call "ANC350_GetSpeed.vi"("error in"=w677, "axis no"=w675, "device handle"=w676) -> ("error out"=w709:T6, "speed"=w698:i32, "device handle"=w710:i32)  [unwired: 2 in]
        n349 = And(x=w673, y=w659) -> (x .and. y?=w665:bool)
        n350 = Select(t=w671, s=w665, f=w672) -> (s? t:f=→"axis 2:\nCurrent position (°)" →"axis 2:\nCurrent position [µm/°/m°] 2":dbl)
        n351 = call "ANC350_GetStepWidth.vi"("error in"=w709, "axis no"=w702, "device handle"=w710) -> ("error out"=w669:T6, "StepWidth"=→"axis 2:\nStepWidth":i32, "device handle"=w667:i32)  [unwired: 2 in]
        n352 = Divide(x=w698, y=1000) -> (x/y=→"axis 2:\nspeed (°/s)":dbl)
        n353 = Divide(x=w707, y=1000) -> (x/y=→"axis 1:\nspeed (°/s)":dbl)
        n354 = And(x=w666, y=w665) -> (x .and. y?=w664:bool)
        n355 = Or(x=w663, y=w662) -> (x .or. y?=w661:bool)
        n356 = case shown="True" w664 {
          tunnel: w669 -> [w729 w733]
          tunnel: [w729 w732] -> w668
          tunnel: w667 -> [_ w731]
          frame False {
          }
          frame True {
            w730 = 1 ("static amplitude")
            n357 = local write "static amplitude (mV)"(w730) -> ()
            n358 = call "ANC350_StaticAmplitude.vi"("error in"=w733, "static amplitude"=w730, "device handle"=w731) -> ("error out"=w732:T6)  [unwired: 3 in, 1 out]
          }
        }
        n359 = case shown="True" w661 {
          frame False {
            # "output timeout"
            n360 = local read "last move time"() -> (w725:timestamp)
            n361 = Get Date/Time In Seconds() -> (seconds since 1Jan1904=w726:timestamp)
            n362 = Subtract(x=w726, y=w725) -> (x-y=w724:dbl)
            n363 = Greater?(x=w724, y=1800.0) -> (0:w722:bool)
            n364 = case shown="True" w722 {
              frame False {
              }
              frame True {
                n365 = property on="both axes: Output" class="Bool (strict)"("Val(Sgnl)"=FALSE ("Value (Signaling)")) -> ()  [unwired: 2 in, 2 out]
              }
            }
          }
          frame True {
            n366 = Get Date/Time In Seconds() -> (seconds since 1Jan1904=w728:timestamp)
            n367 = local write "last move time"(w728) -> ()
          }
        }
        n368 = call <vilib>:"Add State(s) to Queue__JKI_lib_State_Machine.vi"("State(s) in (\"\")"=w721) -> ("States Out"=w720:string)  [unwired: 14 in]
      }
      frame "Attocube: Log to DSC" {
        n369 = local read "axis 1:\nCurrent position (°)"() -> (w747:dbl)
        n370 = local read "axis 1:\npositioner status"() -> (w739:T1)
        n371 = local read "axis 1:\nFrequency [Hz]"() -> (w777:i32)
        n372 = local read "axis 1:\nAmplitude [V]"() -> (w737:dbl)
        n373 = local read "axis 1:\ncontrol mode"() -> (w776:enum16{"speed", "amplitude", "step size"})
        n374 = local read "axis 1:\nsp position °"() -> (w775:dbl)
        n375 = local read "axis 1:\nCapacitance"() -> (w779:i32)
        n376 = local read "axis 1:\nsp rot count"() -> (w774:i32)
        n377 = local read "axis 1:\nDCLevel [V]"() -> (w778:dbl)
        n378 = local read "axis 1:\nspeed (°/s)"() -> (w741:i32)
        n379 = local read "axis 1:\nStepWidth"() -> (w743:i32)
        n380 = local read "axis 1:\nrot. count"() -> (w745:i32)
        n381 = local read "axis 1:\nSingle Circle Mode"() -> (w763:bool)
        n382 = local read "axis 1:\nstop detection"() -> (w758:bool)
        n383 = Unbundle By Name(w739) -> ("moving"=w762:bool, "stop detected"=w761:bool, "sensor error"=w760:bool, "sensor disconnected"=w759:bool)
        n384 = local read "axis 1: \nTarget GND"() -> (w765:bool)
        n385 = local read "axis 1:\nOutput"() -> (w764:bool)
        n386 = Build Array(w737, w779, w747, w778, w777, w743, w776, w745, w775, w774, w741) -> (w767:dbl[])
        n387 = local read "axis 2:\nCurrent position (°)"() -> (w746:dbl)
        n388 = local read "static amplitude (mV)"() -> (w734:dbl)
        n389 = local read "axis 2:\nFrequency [Hz]"() -> (w771:i32)
        n390 = local read "axis 2:\nAmplitude [V]"() -> (w736:dbl)
        n391 = local read "axis 2:\ncontrol mode"() -> (w770:enum16{"speed", "amplitude", "step size"})
        n392 = local read "axis 2:\nsp position °"() -> (w769:dbl)
        n393 = local read "axis 2:\nCapacitance"() -> (w773:i32)
        n394 = local read "axis 2:\nsp rot count"() -> (w768:i32)
        n395 = local read "axis 2:\nDCLevel [V]"() -> (w772:dbl)
        n396 = local read "axis 2:\nspeed (°/s)"() -> (w740:i32)
        n397 = local read "axis 2:\nStepWidth"() -> (w742:i32)
        n398 = local read "axis 2:\nrot. count"() -> (w744:i32)
        n399 = Build Array(w765, w764, w763, w762, w761, w760, w759, w758) -> (w757:bool[])
        n400 = local read "axis 2:\npositioner status"() -> (w738:T1)
        n401 = Build Array (concatenate)(w767, w736, w773, w746, w772, w771, w742, w770, w744, w769, w768, w740, w734) -> (w766:dbl[])
        n402 = local read "axis 2:\nSingle Circle Mode"() -> (w754:bool)
        n403 = local read "axis 2:\nstop detection"() -> (w749:bool)
        n404 = Unbundle By Name(w738) -> ("moving"=w753:bool, "stop detected"=w752:bool, "sensor error"=w751:bool, "sensor disconnected"=w750:bool)
        n405 = local read "axis 2: \nTarget GND"() -> (w756:bool)
        n406 = local read "axis 2:\nOutput"() -> (w755:bool)
        n407 = Build Array (concatenate)(w757, w756, w755, w754, w753, w752, w751, w750, w749) -> (w748:bool[])
        n408 = call <vilib>:"Add State(s) to Queue__JKI_lib_State_Machine.vi"("State(s) in (\"\")"=w782) -> ("States Out"=w781:string)  [unwired: 14 in]
        n409 = call "Attocube_to_DSC.vi"("boolean"=w748, "dbl"=w766) -> ()  [unwired: 6 in]
      }
      frame "Attocube: FGV" {
        n410 = local read "axis 1:\nStop moving"() -> (w827:bool)
        n411 = local read "axis 2:\nStop moving"() -> (w828:bool)
        n412 = local read "set static amplitude\nwhen moving"() -> (w783:bool)
        n413 = local read "axis 1:\nAbsolute"() -> (w825:bool)
        n414 = local read "axis 2:\nAbsolute"() -> (w826:bool)
        n415 = local read "axis 1:\nOutput"() -> (w785:bool)
        n416 = local read "axis 2:\nOutput"() -> (w784:bool)
        n417 = local read "axis 1:\nFrequency [Hz]"() -> (w813:i32)
        n418 = local read "axis 1:\nFrequency [Hz]"() -> (w814:i32)
        n419 = local read "axis 1:\nAmplitude [V]"() -> (w809:dbl)
        n420 = local read "axis 2:\nAmplitude [V]"() -> (w810:dbl)
        n421 = local read "axis 1:\nsp position °"() -> (w815:dbl)
        n422 = local read "axis 2:\nsp position °"() -> (w816:dbl)
        n423 = local read "axis 1:\nsp rot count"() -> (w817:i32)
        n424 = local read "axis 2:\nsp rot count"() -> (w818:i32)
        n425 = local read "axis 1:\nDCLevel [V]"() -> (w811:dbl)
        n426 = local read "axis 2:\nDCLevel [V]"() -> (w812:dbl)
        n427 = call "FGV - Attocube Actions.vi"("error in"=w824, "Function"=enum16{"write", "read"}."read") -> ("error out"=w820:errorcluster, "Actions OUT"=w822:T4)  [unwired: 4 in]
        n428 = Bundle By Name(cluster=w822, "axis 1: Absolute"=w825, "axis 2: Absolute"=w826, "axis 1: Stop moving"=w827, "axis 2: Stop moving"=w828, "axis 1: Output"=w785, "axis 2: Output"=w784, "set static amplitude\nwhen moving"=w783) -> (w821:T4)
        n429 = call "FGV - Attocube Actions.vi"("error in"=w820, "Function"=enum16{"write", "read"}."write", "Actions IN"=w821) -> ("error out"=w808:errorcluster)  [unwired: 3 in, 1 out]
        n430 = call "FGV - Attocube Targets.vi"("error in"=w808, "Function"=enum16{"write", "read"}."read") -> ("error out"=w804:errorcluster, "Targets Out"=w806:T5)  [unwired: 4 in]
        n431 = Bundle By Name(cluster=w806, "axis 1: Amplitude [V]"=w809, "axis 2: Amplitude [V]"=w810, "axis 1: DCLevel [V]"=w811, "axis 2: DCLevel [V]"=w812, "axis 1: Frequency [Hz]"=w813, "axis 2: Frequency [Hz]"=w814, "axis 1: sp position °"=w815, "axis 2: sp position °"=w816, "axis 1: sp rot count"=w817, "axis 2: sp rot count"=w818) -> (w803:T5)
        n432 = local read "axis 1:\nCurrent position (°)"() -> (w793:dbl)
        n433 = local read "axis 2:\nCurrent position (°)"() -> (w794:dbl)
        n434 = call "FGV - Attocube Targets.vi"("error in"=w804, "Function"=enum16{"write", "read"}."write", "Targets In"=w803) -> ("error out"=w792:errorcluster)  [unwired: 3 in, 1 out]
        n435 = local read "axis 1:\npositioner status"() -> (w801:T1)
        n436 = local read "axis 2:\npositioner status"() -> (w802:T1)
        n437 = local read "axis 1:\nspeed (°/s)"() -> (w799:i32)
        n438 = local read "axis 2:\nspeed (°/s)"() -> (w800:i32)
        n439 = local read "axis 1:\nStepWidth"() -> (w797:i32)
        n440 = local read "axis 2:\nStepWidth"() -> (w798:i32)
        n441 = local read "axis 1:\nrot. count"() -> (w795:i32)
        n442 = local read "axis 2:\nrot. count"() -> (w796:i32)
        n443 = call "FGV - Attocube Status.vi"("error in"=w792, "Function"=enum16{"write", "read"}."read") -> ("error out"=w788:errorcluster, "Status OUT"=w790:T9)  [unwired: 4 in]
        n444 = Bundle By Name(cluster=w790, "axis 1: Current position (°)"=w793, "axis 2: Current position (°)"=w794, "axis 1: rot. count"=w795, "axis 2: rot. count"=w796, "axis 1: StepWidth"=w797, "axis 2: StepWidth"=w798, "axis 1: speed (°/s)"=w799, "axis 2: speed (°/s)"=w800, "axis 1: positioner status"=w801, "axis 2: positioner status"=w802) -> (w786:T9)
        n445 = call <vilib>:"Add State(s) to Queue__JKI_lib_State_Machine.vi"("State(s) in (\"\")"=w831) -> ("States Out"=w830:string)  [unwired: 14 in]
        n446 = call "FGV - Attocube Status.vi"("error in"=w788, "Function"=enum16{"write", "read"}."write", "Status IN"=w786) -> ("error out"=w787:errorcluster)  [unwired: 3 in, 1 out]
      }
    }
  }
  n447 = disable-structure shown="Disabled" {
    frame Disabled {
      n448 = call "ANC350_StaticAmplitude.vi"() -> ()  [unwired: 6 in, 2 out]
    }
    frame Enabled {
    }
  }
  n449 = disable-structure shown="Disabled" {
    disable-tunnel: [w833 _] -> _
    disable-tunnel: [w832 _] -> _
    frame Disabled {
      n450 = call "visualize.vi"() -> ("small angle"=w832:sgl, "large axis angle"=w833:sgl)  [unwired: 9 in, 1 out]
    }
    frame Enabled {
    }
  }
